vi "Grid_Monitor_V2backupwhite.vi"(7 "Stop (In)":refnum<notifier>, 8 "Error (In)":errorcluster, 11 "SCADA AugState (In)":refnum<notifier>) -> (0 "Error (Out)":errorcluster, 3 "SCADA AugState (Out)":refnum<notifier>, 6 "Stop (Out)":refnum<notifier>)   [LabVIEW 2021]
uses:
  SCADA/SCADA Augmented State.ctl
  Interval.ctl
  SCADA/SCADA Augmented State GUPTA.ctl
  <vilib>/Utility/miscctls.llb/LVForegroundBackgroundColorsTypeDef.ctl
panel:
  out "kW":dbl caption="Numeric" format="%#.3g"
  out "?VkVAr":dbl caption="Numeric" format="%.3g"
  out "A":dbl[unit] caption="Numeric" format="%-^#10.3g"
  out "kW":dbl caption="Numeric" format="%#.3g"
  out "?VkVAr":dbl caption="Numeric" format="%.3g"
  out "A":dbl[unit] caption="Numeric" format="%-^#10.3g"
  out "kW":dbl caption="Numeric" format="%#.3g"
  out "?VkVAr":dbl caption="Numeric" format="%.3g"
  out "A":dbl[unit] caption="Numeric" format="%-^#10.3g"
  out "kW":dbl caption="Numeric" format="%#.3g"
  out "?VkVAr":dbl caption="Numeric" format="%.3g"
  out "A":dbl[unit] caption="Numeric" format="%-^#10.3g"
  out "kW":dbl caption="Numeric" format="%#.3g"
  out "?VkVAr":dbl caption="Numeric" format="%.3g"
  out "A":dbl[unit] caption="Numeric" format="%-^#10.3g"
  out "kW":dbl caption="Numeric" format="%#.3g"
  out "?VkVAr":dbl caption="Numeric" format="%.3g"
  out "A":dbl[unit] caption="Numeric" format="%-^#10.3g"
  out "kW":dbl caption="Numeric" format="%#.3g"
  out "?VkVAr":dbl caption="Numeric" format="%.3g"
  out "A":dbl[unit] caption="Numeric" format="%-^#10.3g"
  out "kW":dbl caption="Numeric" format="%#.3g"
  out "?VkVAr":dbl caption="Numeric" format="%.3g"
  out "A":dbl[unit] caption="Numeric" format="%-^#10.3g"
  out "A":dbl caption="Numeric" format="%-^#10.3g"
  out "kW":dbl caption="Numeric" format="%#.3g"
  out "A":dbl caption="Numeric" format="%-^#10.3g"
  out "kW":dbl caption="Numeric" format="%#.3g"
  out "A":dbl caption="Numeric" format="%-^#10.3g"
  out "kW":dbl caption="Numeric" format="%#.3g"
  out "A":dbl caption="Numeric" format="%-^#10.3g"
  out "kW":dbl caption="Numeric" format="%#.3g"
  out "V slider 11":T1(slide) caption="V-i" scale=230.0..240.0 scale format="%#_4g"
  out "V slider 25":dbl(slide) caption="V-i" max=-10.0 scale=720.0..750.0 scale format="%#_4g"
  out "V slider 24":dbl(slide) caption="V-i" max=-10.0 scale=720.0..750.0 scale format="%#_4g"
  out "V slider 23":dbl(slide) caption="V-i" max=-10.0 scale=720.0..750.0 scale format="%#_4g"
  out "V slider 22":dbl(slide) caption="V-i" max=-10.0 scale=720.0..750.0 scale format="%#_4g"
  out "V slider 21":dbl(slide) caption="V-i" max=-10.0 scale=720.0..750.0 scale format="%#_4g"
  out "V slider 20":dbl(slide) caption="V-i" max=-10.0 scale=720.0..750.0 scale format="%#_4g"
  out "V slider 19":dbl(slide) caption="V-i" max=-10.0 scale=720.0..750.0 scale format="%#_4g"
  out "V slider 18":dbl(slide) caption="V-i" max=-10.0 scale=720.0..750.0 scale format="%#_4g"
  out "V slider 17":T1(slide) caption="V-i" scale=230.0..240.0 scale format="%#_4g"
  out "V slider 16":T1(slide) caption="V-i" scale=230.0..240.0 scale format="%#_4g"
  out "V slider 15":T1(slide) caption="V-i" scale=230.0..240.0 scale format="%#_4g"
  out "V slider 14":T1(slide) caption="V-i" scale=230.0..240.0 scale format="%#_4g"
  out "V slider 13":T1(slide) caption="V-i" scale=230.0..240.0 scale format="%#_4g"
  out "V slider 12":T1(slide) caption="V-i" scale=230.0..240.0 scale format="%#_4g"
  out "V slider 10":T1(slide) caption="V-i" scale=230.0..240.0 scale format="%#_4g"
  out "V slider 9":T1(slide) caption="V-i" scale=230.0..240.0 scale format="%#_4g"
  out "V slider 8":T1(slide) caption="V-i" scale=230.0..240.0 scale format="%#_4g"
  out "V slider 7":T1(slide) caption="V-i" scale=230.0..240.0 scale format="%#_4g"
  out "V slider 6":T1(slide) caption="V-i" scale=230.0..240.0 scale format="%#_4g"
  out "V slider 4":T1(slide) caption="V-i" scale=230.0..240.0 scale format="%#_4g"
  out "V slider 3":T1(slide) caption="V-i" scale=230.0..240.0 scale format="%#_4g"
  out "V slider 1":T1(slide) caption="V-i" scale=230.0..240.0 scale format="%#_4g"
  out "V slider 0":T1(slide) caption="V-i" scale=230.0..240.0 scale format="%#_4g"
  out "I slider 20":dbl(slide) min=-10.0 max=100.0 scale=0.0..100.0
  out "I slider 19":dbl(slide) min=-10.0 max=100.0 scale=0.0..100.0
  out "I slider 18":dbl(slide) min=-10.0 max=100.0 scale=0.0..100.0
  out "I slider 17":dbl(slide) min=-10.0 max=100.0 scale=0.0..100.0
  out "I slider 16":T1(slide) scale=0.0..44.0
  out "I slider 15":T1(slide) scale=0.0..44.0
  out "I slider 14":T1(slide) scale=0.0..44.0
  out "I slider 13":T1(slide) scale=0.0..44.0
  out "I slider 12":T1(slide) scale=0.0..108.0
  out "I slider 11":T1(slide) scale=0.0..82.0
  out "I slider 10":T1(slide) scale=0.0..82.0 scale format="%^#1.3g"
  out "I slider 9":T1(slide) scale=0.0..44.0
  out "I slider 8":T1(slide) scale=0.0..82.0 scale format="%^#1.3g"
  out "I slider 7":T1(slide) scale=0.0..207.0
  out "I slider 6":T1(slide) scale=0.0..135.0 scale format="%^#1.3g"
  out "I slider 5":T1(slide) scale=0.0..82.0
  out "I slider 4":T1(slide) scale=0.0..82.0
  out "I slider 3":T1(slide) scale=0.0..108.0
  out "I slider 2":T1(slide) scale=0.0..207.0 scale format="%^#1.3g"
  out "I slider 0":T1(slide) scale=0.0..207.0
  out "I slider 1":T1(slide) scale=0.0..44.0
  out "V slider 2":T1(slide) caption="V-i" scale=230.0..240.0 scale format="%#_4g"
  out "A":dbl caption="Numeric" format="%-^#10.3g"
  out "kW":dbl caption="Numeric" format="%#.3g"
  out "A":dbl caption="Numeric" format="%-^#10.3g"
  out "kW":dbl caption="Numeric" format="%#.3g"
  out "A":dbl caption="Numeric" format="%-^#10.3g"
  out "kW":dbl caption="Numeric" format="%#.3g"
  out "A":dbl[unit] caption="Numeric" format="%-^#10.3g"
  out "?VkVAr":dbl caption="Numeric" format="%.3g"
  out "kW":dbl caption="Numeric" format="%#.3g"
  out "A":dbl[unit] caption="Numeric" format="%-^#10.3g"
  out "?VkVAr":dbl caption="Numeric" format="%.3g"
  out "kW":dbl caption="Numeric" format="%#.3g"
  in  "Stop?":bool
  out "Connected?":bool
  out "AugState (Out)":refnum<notifier>
  in  "AugState (In)":refnum<notifier>
  # "EL"
  # "L"
  # "Electrolyzer"
  # "Load"
  # "FC"
  # "B"
  # "Fuel Cell"
  # "Battery"
  # "PV"
  # "SC"
  # "Photovoltaic"
  # "Super Caps"
  # "V"
  # "B03"
  # "B01"
  # "PMU locations"
  # "DMU locations"
  # "B02"
  # "1"
  # "9"
  # "2"
  # "B05"
  # "B07"
  # "B14"
  # "B04"
  # "B06"
  # "7"
  # "3"
  # "A"
  # "B18"
  # "B22"
  # "B26"
  # "4"
  # "8"
  # "10"
  # "A"
  # "B09"
  # "B08"
  # "B17"
  # "B21"
  # "B25"
  # "4"
  # "3"
  # "7"
  # "11"
  # "B11"
  # "B16"
  # "B20"
  # "B24"
  # "B10"
  # "5"
  # "2"
  # "6"
  # "12"
  # "B13"
  # "B12"
  # "6"
  # "B15"
  # "B19"
  # "B23"
  # "1"
  # "5"
  # "13"
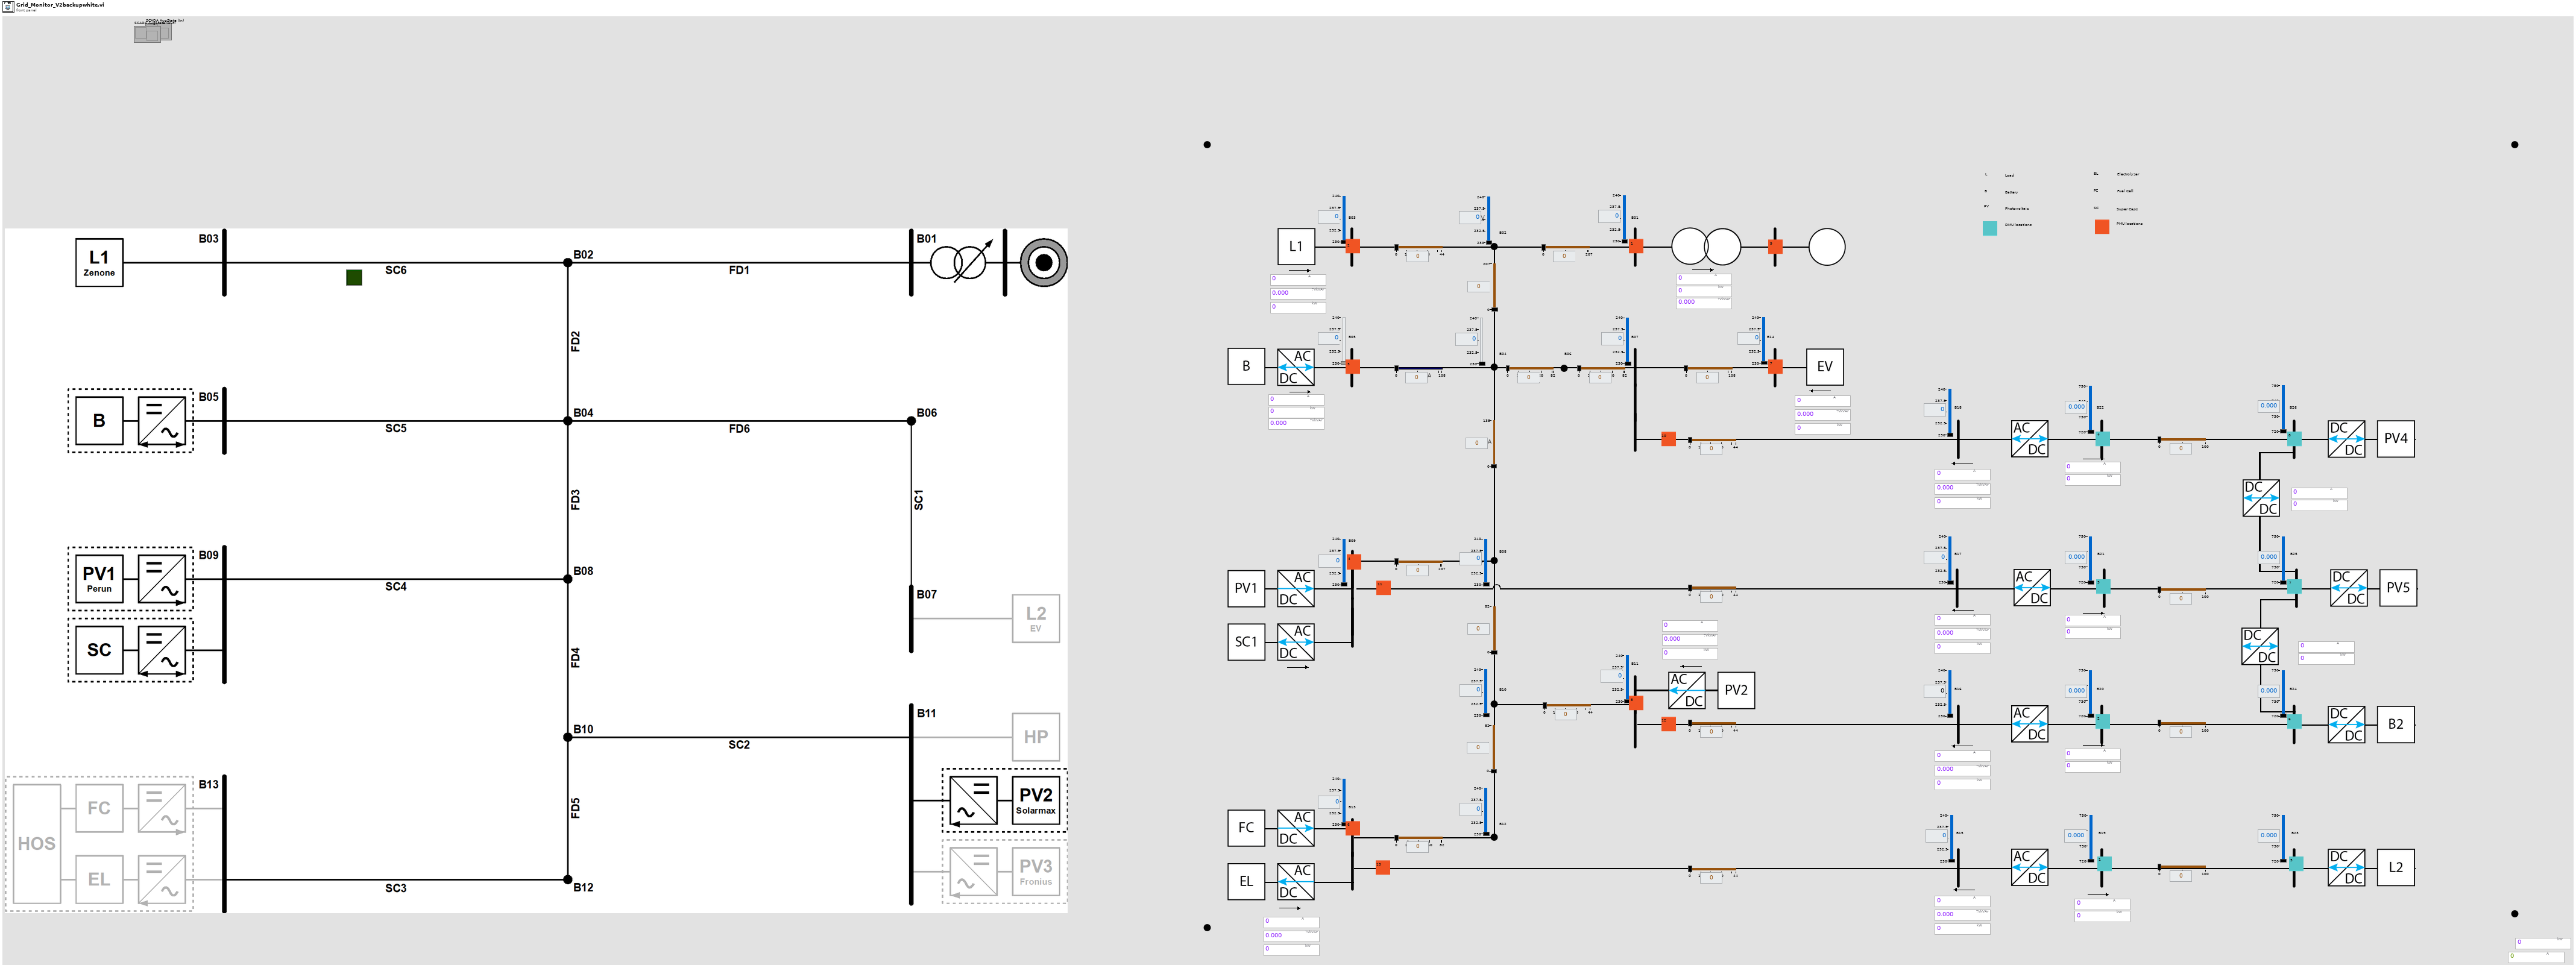
[diagram p1: front panel]
types:
  T1 = cluster{"Numeric":dbl, "Numeric":dbl, "Numeric":dbl}
  T2 = typedef "LVForegroundBackgroundColorsTypeDef.ctl" = cluster{"Foreground Color":u32, "Background Color":u32}
  T3 = typedef "SCADA Augmented State GUPTA.ctl" = cluster{"Buses":cluster{"Vbus":cdb[], "Iinjected":cdb[], "Sinjected":cdb[], "Vband":T4}[], "Lines":cluster{"Iforward":cdb[], "Ibackward":cdb[], "Imaximum":dbl}[], "f_downstream":dbl, "V_upstream":cdb[], "f_upstream":dbl, "Timestamp":timestamp, "M ":cluster{cdb, cdb, cdb}[], "z(k|k)":dbl[], "r(k)":dbl[], "Arrival (SE)":timestamp, "Arrival (PDC)":timestamp, "Departure (SE)":timestamp, "T":dbl[]}
  T4 = typedef "Interval.ctl" = cluster{"lower":dbl, "upper":dbl}
  T5 = cluster{"Iforward":cdb[], "Ibackward":cdb[], "Imaximum":dbl}[]
  T6 = cluster{"Vbus":cdb[], "Iinjected":cdb[], "Sinjected":cdb[], "Vband":T4}[]
  T7 = cluster{"Vbus":cdb[], "Iinjected":cdb[], "Sinjected":cdb[], "Vband":T4}
  T8 = cluster{"I_trip":dbl, "Phasor C":dbl, "Phasor C":dbl, "Phasor C":dbl}
  T9 = cluster{"V_maximum":dbl, "Phasor C":dbl, "Phasor C":dbl, "Phasor C":dbl, "V_minimun":dbl}
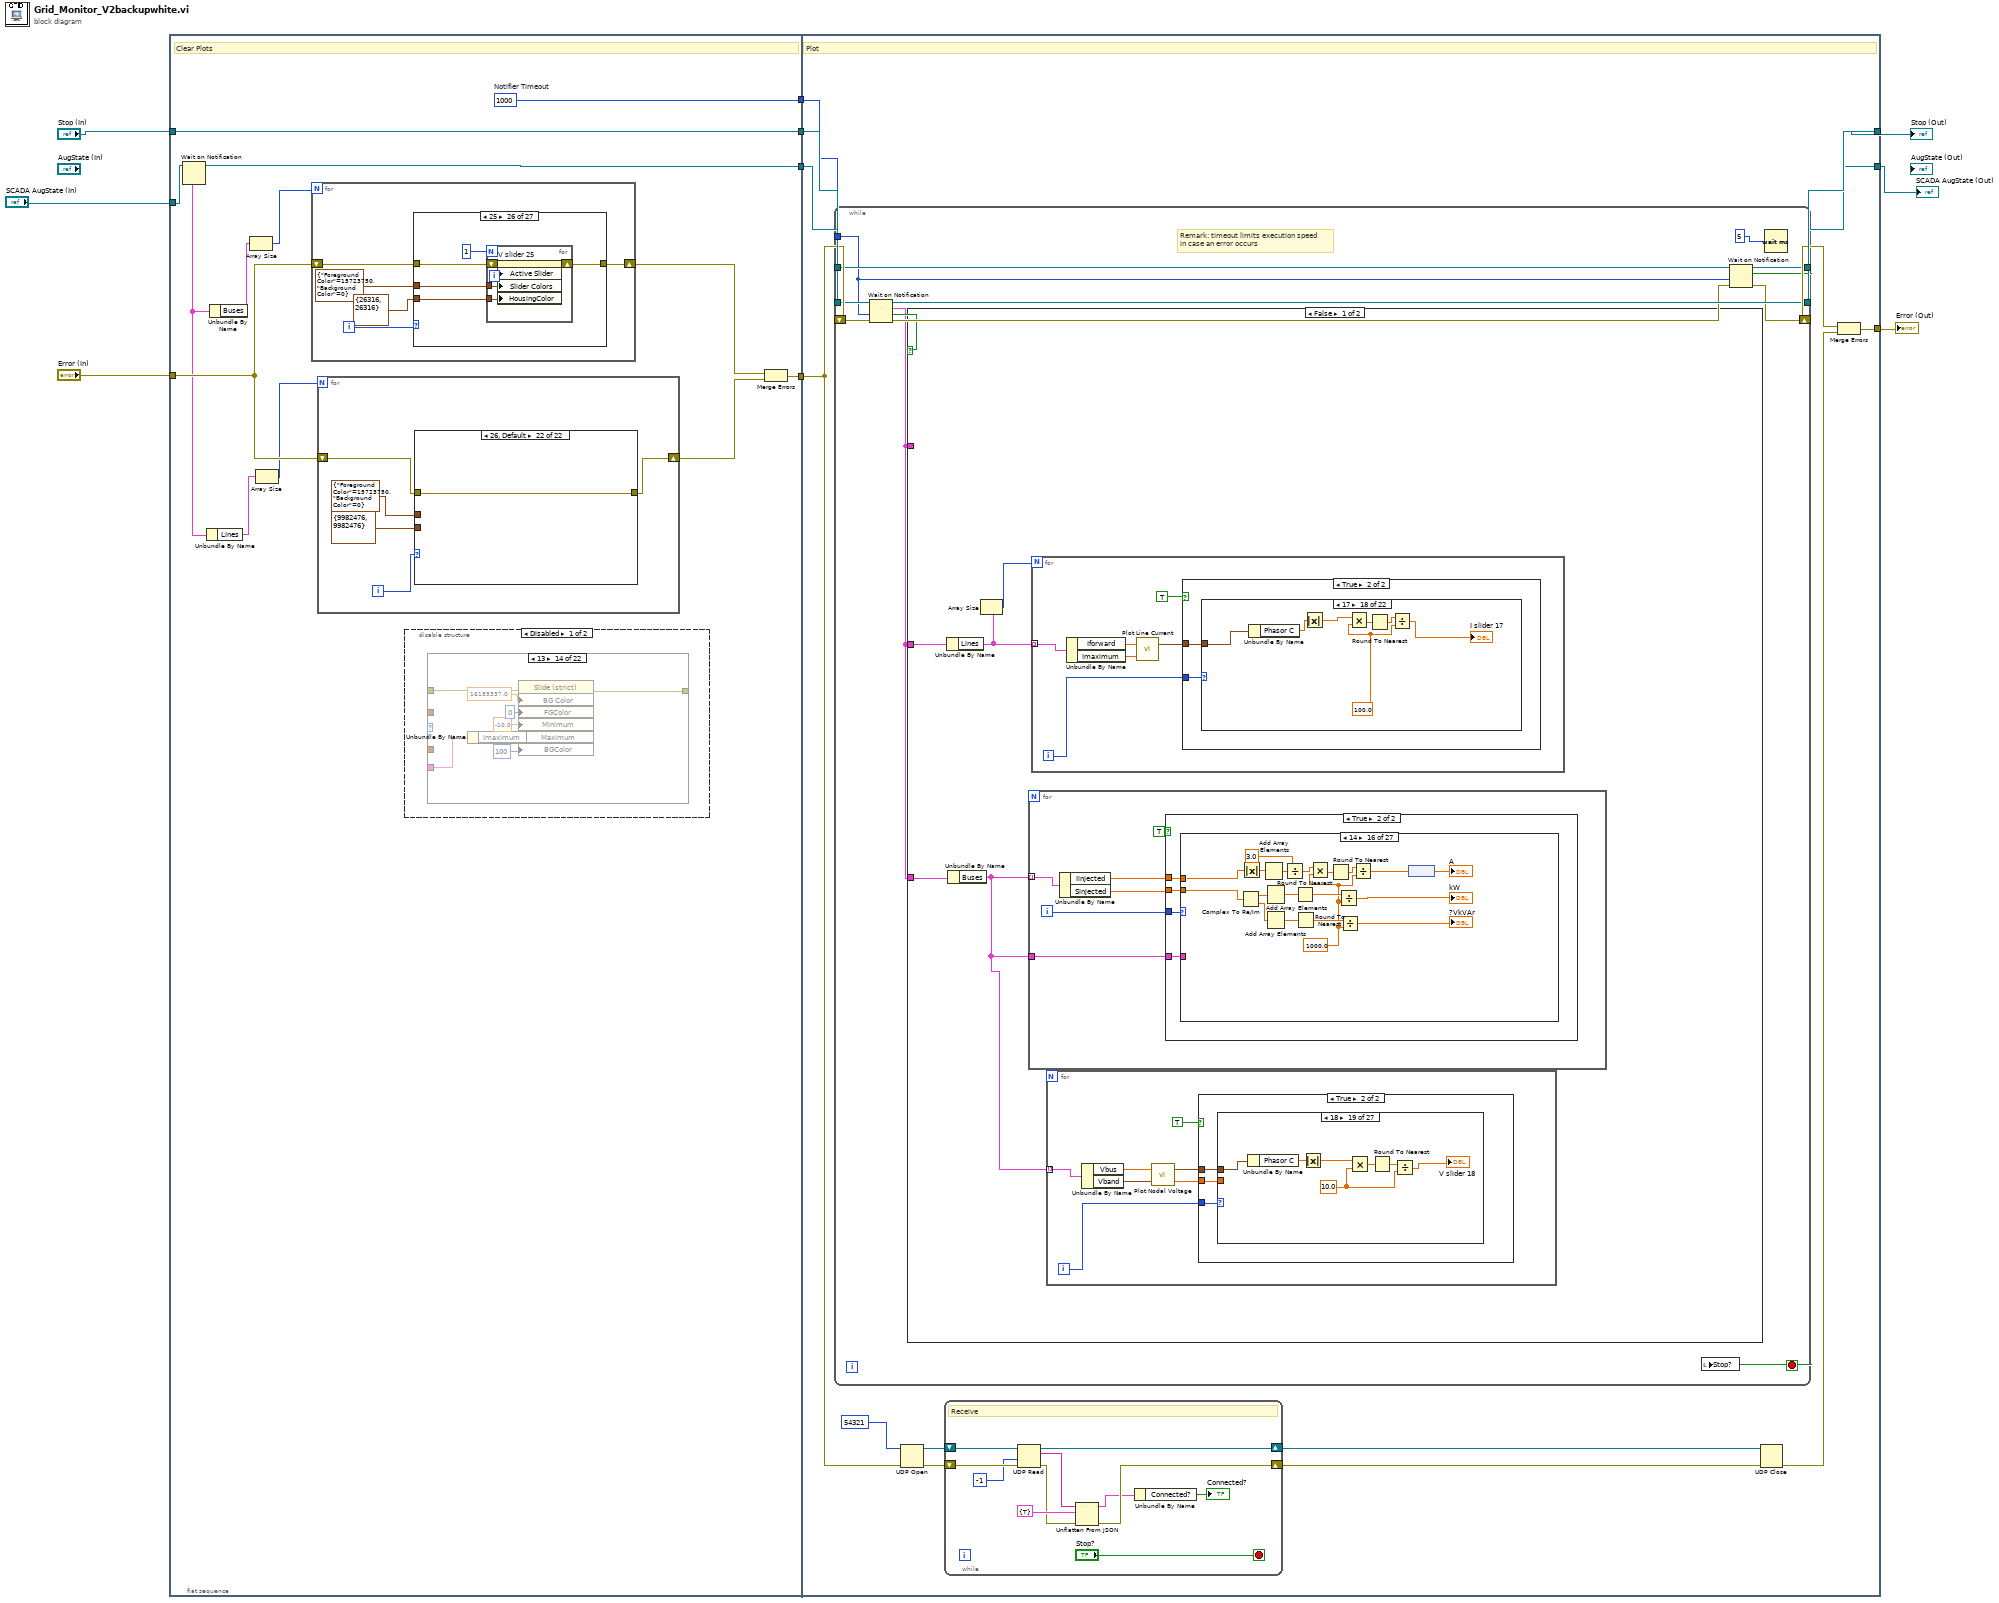
[diagram p0: block diagram]
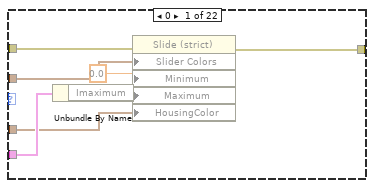
[diagram p2: hidden frame]
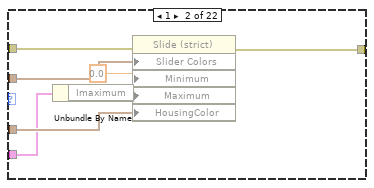
[diagram p3: hidden frame]
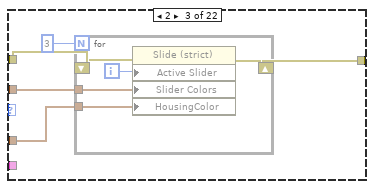
[diagram p4: hidden frame]
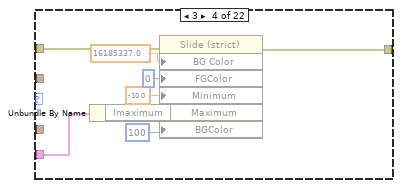
[diagram p5: hidden frame]
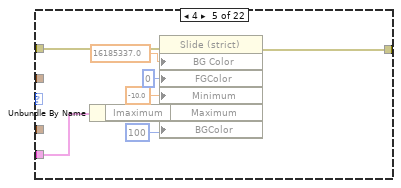
[diagram p6: hidden frame]
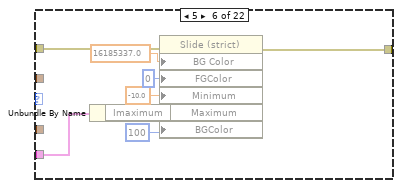
[diagram p7: hidden frame]
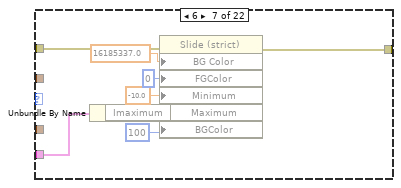
[diagram p8: hidden frame]
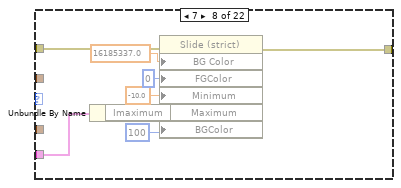
[diagram p9: hidden frame]
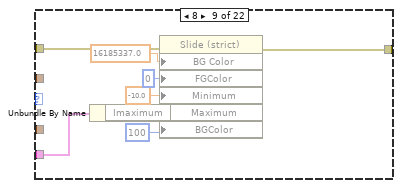
[diagram p10: hidden frame]
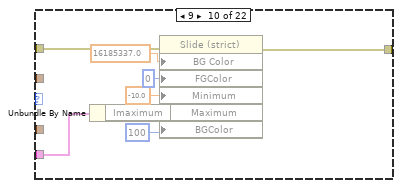
[diagram p11: hidden frame]
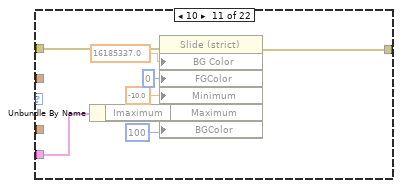
[diagram p12: hidden frame]
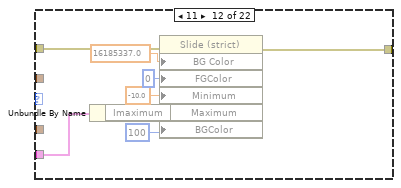
[diagram p13: hidden frame]
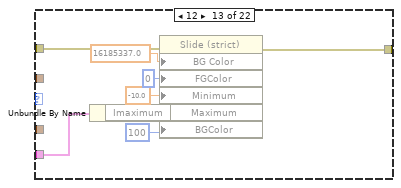
[diagram p14: hidden frame]
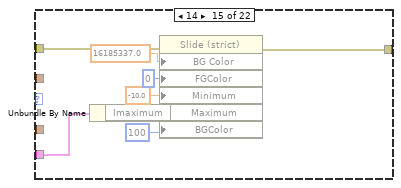
[diagram p15: hidden frame]
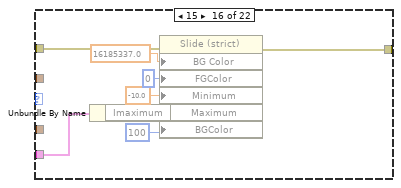
[diagram p16: hidden frame]
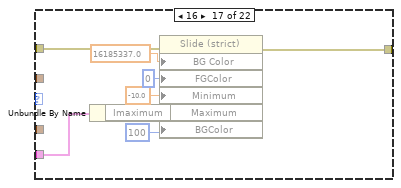
[diagram p17: hidden frame]
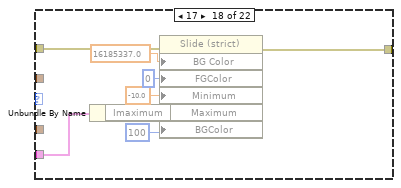
[diagram p18: hidden frame]
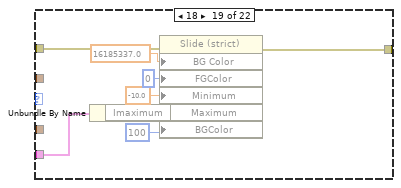
[diagram p19: hidden frame]
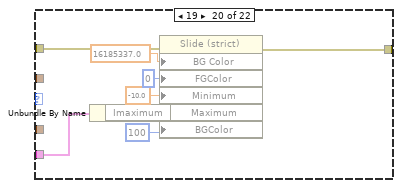
[diagram p20: hidden frame]
diagram:
  n1 = flat-sequence {
    tunnel: "Stop (In)" -> [w23]
    tunnel: [w16] -> w8
    tunnel: [w23] -> w7
    tunnel: [w20] -> w6
    tunnel: "Error (In)" -> [w19]
    tunnel: [w18] -> w3
    tunnel: "SCADA AugState (In)" -> [w17]
    tunnel: [w677] -> w9
    tunnel: [w668] -> w4
    tunnel: w8 -> [w679]
    tunnel: w7 -> [w678]
    tunnel: w6 -> [w670]
    tunnel: w3 -> [w676]
    tunnel: [w666] -> w2
    frame #0 {
      w18 = 1000  # Notifier Timeout
      # "Clear Plots"
      n2 = Wait on Notification(notifier=w17) -> (notifier out=w16:refnum<notifier>, notification=w14:T3)  [unwired: 3 in, 2 out]
      n3 = Unbundle By Name(w14) -> ("Lines"=w11:T5)
      n4 = Unbundle By Name(w14) -> ("Buses"=w13:T6)
      n5 = Array Size(array=w13) -> (size(s)=w12:i32)
      n6 = Array Size(array=w11) -> (size(s)=w15:i32)
      n7 = for {
        N: w12 -> [_]
        shift-right: [w409] -> w22
        shift-left: w19 -> [w411]
        i -> [w410]
        n8 = case shown="25" w410 {
          tunnel: w411 -> [w415 w425 w435 w444 w453 w462 w468 w478 w488 w498 w508 w518 w528 w538 w548 w558 w568 w578 w588 w598 w608 w618 w628 w638 w648 w658 w665]
          tunnel: [w416 w426 w436 w445 w454 w463 w469 w479 w489 w499 w509 w519 w529 w539 w549 w559 w569 w579 w589 w599 w609 w619 w629 w639 w649 w659 w665] -> w409
          tunnel: T2 {"Foreground Color"=15723750, "Background Color"=0} ("Slider Colors") -> [w413 w423 w433 w442 w451 w460 w466 w476 w486 w496 w506 w516 w526 w536 w546 w556 w566 w576 w586 w596 w606 w616 w626 w636 w646 w656 _]
          tunnel: T2 {"Foreground Color"=26316, "Background Color"=26316} ("Slider Colors") -> [w412 w422 w432 _ w450 _ w465 w475 w485 w495 w505 w515 w525 w535 w545 w555 w565 w575 w585 w595 w605 w615 w625 w635 w645 w655 _]
          frame 0 {
            n9 = for {
              N: 3 -> [_]
              tunnel: w413 -> [w419]
              shift-right: [w421] -> w416
              shift-left: w415 -> [w420]
              tunnel: w412 -> [w417]
              i -> [w418]
              n10 = property on="V slider 0" class="Slide (strict)"(error in=w420, "Active Slider"=w418, "Slider Colors"=w419, "HousingColor"=w417) -> (error out=w421:errorcluster)  [unwired: 1 in, 1 out]
            }
          }
          frame 1 {
            n11 = for {
              N: 3 -> [_]
              tunnel: w423 -> [w429]
              shift-right: [w431] -> w426
              shift-left: w425 -> [w430]
              tunnel: w422 -> [w427]
              i -> [w428]
              n12 = property on="V slider 1" class="Slide (strict)"(error in=w430, "Active Slider"=w428, "Slider Colors"=w429, "HousingColor"=w427) -> (error out=w431:errorcluster)  [unwired: 1 in, 1 out]
            }
          }
          frame 2 {
            n13 = for {
              N: 3 -> [_]
              tunnel: w433 -> [w439]
              shift-right: [w441] -> w436
              shift-left: w435 -> [w440]
              tunnel: w432 -> [w437]
              i -> [w438]
              n14 = property on="V slider 2" class="Slide (strict)"(error in=w440, "Active Slider"=w438, "Slider Colors"=w439, "HousingColor"=w437) -> (error out=w441:errorcluster)  [unwired: 1 in, 1 out]
            }
          }
          frame 3 {
            n15 = for {
              N: 3 -> [_]
              tunnel: w442 -> [w447]
              shift-right: [w449] -> w445
              shift-left: w444 -> [w448]
              i -> [w446]
              n16 = property on="V slider 3" class="Slide (strict)"(error in=w448, "Active Slider"=w446, "Slider Colors"=w447) -> (error out=w449:errorcluster)  [unwired: 1 in, 1 out]
            }
          }
          frame 4 {
            n17 = for {
              N: 3 -> [_]
              tunnel: w451 -> [w457]
              shift-right: [w459] -> w454
              shift-left: w453 -> [w458]
              tunnel: w450 -> [w455]
              i -> [w456]
              n18 = property on="I slider 4" class="Slide (strict)"(error in=w458, "Active Slider"=w456, "Slider Colors"=w457, "HousingColor"=w455) -> (error out=w459:errorcluster)  [unwired: 1 in, 1 out]
            }
          }
          frame 5 {
            n19 = for {
              N: 3 -> [_]
              tunnel: w460 -> [_]
              shift-right: [w464] -> w463
              shift-left: w462 -> [w464]
            }
          }
          frame 6 {
            n20 = for {
              N: 3 -> [_]
              tunnel: w466 -> [w472]
              shift-right: [w474] -> w469
              shift-left: w468 -> [w473]
              tunnel: w465 -> [w470]
              i -> [w471]
              n21 = property on="V slider 6" class="Slide (strict)"(error in=w473, "Active Slider"=w471, "Slider Colors"=w472, "HousingColor"=w470) -> (error out=w474:errorcluster)  [unwired: 1 in, 1 out]
            }
          }
          frame 7 {
            n22 = for {
              N: 3 -> [_]
              tunnel: w476 -> [w482]
              shift-right: [w484] -> w479
              shift-left: w478 -> [w483]
              tunnel: w475 -> [w480]
              i -> [w481]
              n23 = property on="V slider 7" class="Slide (strict)"(error in=w483, "Active Slider"=w481, "Slider Colors"=w482, "HousingColor"=w480) -> (error out=w484:errorcluster)  [unwired: 1 in, 1 out]
            }
          }
          frame 8 {
            n24 = for {
              N: 3 -> [_]
              tunnel: w486 -> [w492]
              shift-right: [w494] -> w489
              shift-left: w488 -> [w493]
              tunnel: w485 -> [w490]
              i -> [w491]
              n25 = property on="V slider 8" class="Slide (strict)"(error in=w493, "Active Slider"=w491, "Slider Colors"=w492, "HousingColor"=w490) -> (error out=w494:errorcluster)  [unwired: 1 in, 1 out]
            }
          }
          frame 9 {
            n26 = for {
              N: 3 -> [_]
              tunnel: w496 -> [w502]
              shift-right: [w504] -> w499
              shift-left: w498 -> [w503]
              tunnel: w495 -> [w500]
              i -> [w501]
              n27 = property on="V slider 9" class="Slide (strict)"(error in=w503, "Active Slider"=w501, "Slider Colors"=w502, "HousingColor"=w500) -> (error out=w504:errorcluster)  [unwired: 1 in, 1 out]
            }
          }
          frame 10 {
            n28 = for {
              N: 3 -> [_]
              tunnel: w506 -> [w512]
              shift-right: [w514] -> w509
              shift-left: w508 -> [w513]
              tunnel: w505 -> [w510]
              i -> [w511]
              n29 = property on="V slider 10" class="Slide (strict)"(error in=w513, "Active Slider"=w511, "Slider Colors"=w512, "HousingColor"=w510) -> (error out=w514:errorcluster)  [unwired: 1 in, 1 out]
            }
          }
          frame 11 {
            n30 = for {
              N: 3 -> [_]
              tunnel: w516 -> [w521]
              shift-right: [w523] -> w519
              shift-left: w518 -> [w524]
              tunnel: w515 -> [w520]
              i -> [w522]
              n31 = property on="V slider 11" class="Slide (strict)"(error in=w524, "Active Slider"=w522, "Slider Colors"=w521, "HousingColor"=w520) -> (error out=w523:errorcluster)  [unwired: 1 in, 1 out]
            }
          }
          frame 12 {
            n32 = for {
              N: 3 -> [_]
              tunnel: w526 -> [w532]
              shift-right: [w534] -> w529
              shift-left: w528 -> [w533]
              tunnel: w525 -> [w530]
              i -> [w531]
              n33 = property on="V slider 12" class="Slide (strict)"(error in=w533, "Active Slider"=w531, "Slider Colors"=w532, "HousingColor"=w530) -> (error out=w534:errorcluster)  [unwired: 1 in, 1 out]
            }
          }
          frame 13 {
            n34 = for {
              N: 3 -> [_]
              tunnel: w536 -> [w542]
              shift-right: [w544] -> w539
              shift-left: w538 -> [w543]
              tunnel: w535 -> [w540]
              i -> [w541]
              n35 = property on="V slider 13" class="Slide (strict)"(error in=w543, "Active Slider"=w541, "Slider Colors"=w542, "HousingColor"=w540) -> (error out=w544:errorcluster)  [unwired: 1 in, 1 out]
            }
          }
          frame 14 {
            n36 = for {
              N: 3 -> [_]
              tunnel: w546 -> [w552]
              shift-right: [w554] -> w549
              shift-left: w548 -> [w553]
              tunnel: w545 -> [w550]
              i -> [w551]
              n37 = property on="V slider 14" class="Slide (strict)"(error in=w553, "Active Slider"=w551, "Slider Colors"=w552, "HousingColor"=w550) -> (error out=w554:errorcluster)  [unwired: 1 in, 1 out]
            }
          }
          frame 15 {
            n38 = for {
              N: 3 -> [_]
              tunnel: w556 -> [w562]
              shift-right: [w564] -> w559
              shift-left: w558 -> [w563]
              tunnel: w555 -> [w560]
              i -> [w561]
              n39 = property on="V slider 15" class="Slide (strict)"(error in=w563, "Active Slider"=w561, "Slider Colors"=w562, "HousingColor"=w560) -> (error out=w564:errorcluster)  [unwired: 1 in, 1 out]
            }
          }
          frame 16 {
            n40 = for {
              N: 3 -> [_]
              tunnel: w566 -> [w572]
              shift-right: [w574] -> w569
              shift-left: w568 -> [w573]
              tunnel: w565 -> [w570]
              i -> [w571]
              n41 = property on="V slider 16" class="Slide (strict)"(error in=w573, "Active Slider"=w571, "Slider Colors"=w572, "HousingColor"=w570) -> (error out=w574:errorcluster)  [unwired: 1 in, 1 out]
            }
          }
          frame 17 {
            n42 = for {
              N: 3 -> [_]
              tunnel: w576 -> [w582]
              shift-right: [w584] -> w579
              shift-left: w578 -> [w583]
              tunnel: w575 -> [w580]
              i -> [w581]
              n43 = property on="V slider 17" class="Slide (strict)"(error in=w583, "Active Slider"=w581, "Slider Colors"=w582, "HousingColor"=w580) -> (error out=w584:errorcluster)  [unwired: 1 in, 1 out]
            }
          }
          frame 18 {
            n44 = for {
              N: 1 -> [_]
              shift-right: [w594] -> w589
              shift-left: w588 -> [w593]
              tunnel: w586 -> [w591]
              tunnel: w585 -> [w590]
              i -> [w592]
              n45 = property on="V slider 18" class="Slide (strict)"(error in=w593, "Active Slider"=w592, "Slider Colors"=w591, "HousingColor"=w590) -> (error out=w594:errorcluster)  [unwired: 1 in, 1 out]
            }
          }
          frame 19 {
            n46 = for {
              N: 1 -> [_]
              tunnel: w596 -> [w602]
              shift-right: [w604] -> w599
              shift-left: w598 -> [w603]
              tunnel: w595 -> [w600]
              i -> [w601]
              n47 = property on="V slider 19" class="Slide (strict)"(error in=w603, "Active Slider"=w601, "Slider Colors"=w602, "HousingColor"=w600) -> (error out=w604:errorcluster)  [unwired: 1 in, 1 out]
            }
          }
          frame 20 {
            n48 = for {
              N: 1 -> [_]
              tunnel: w606 -> [w612]
              shift-right: [w614] -> w609
              shift-left: w608 -> [w613]
              tunnel: w605 -> [w610]
              i -> [w611]
              n49 = property on="V slider 20" class="Slide (strict)"(error in=w613, "Active Slider"=w611, "Slider Colors"=w612, "HousingColor"=w610) -> (error out=w614:errorcluster)  [unwired: 1 in, 1 out]
            }
          }
          frame 21 {
            n50 = for {
              N: 1 -> [_]
              tunnel: w616 -> [w622]
              shift-right: [w624] -> w619
              shift-left: w618 -> [w623]
              tunnel: w615 -> [w620]
              i -> [w621]
              n51 = property on="V slider 21" class="Slide (strict)"(error in=w623, "Active Slider"=w621, "Slider Colors"=w622, "HousingColor"=w620) -> (error out=w624:errorcluster)  [unwired: 1 in, 1 out]
            }
          }
          frame 22 {
            n52 = for {
              N: 1 -> [_]
              tunnel: w626 -> [w632]
              shift-right: [w634] -> w629
              shift-left: w628 -> [w633]
              tunnel: w625 -> [w630]
              i -> [w631]
              n53 = property on="V slider 22" class="Slide (strict)"(error in=w633, "Active Slider"=w631, "Slider Colors"=w632, "HousingColor"=w630) -> (error out=w634:errorcluster)  [unwired: 1 in, 1 out]
            }
          }
          frame 23 {
            n54 = for {
              N: 1 -> [_]
              tunnel: w636 -> [w642]
              shift-right: [w644] -> w639
              shift-left: w638 -> [w643]
              tunnel: w635 -> [w640]
              i -> [w641]
              n55 = property on="V slider 23" class="Slide (strict)"(error in=w643, "Active Slider"=w641, "Slider Colors"=w642, "HousingColor"=w640) -> (error out=w644:errorcluster)  [unwired: 1 in, 1 out]
            }
          }
          frame 24 {
            n56 = for {
              N: 1 -> [_]
              tunnel: w646 -> [w652]
              shift-right: [w654] -> w649
              shift-left: w648 -> [w653]
              tunnel: w645 -> [w650]
              i -> [w651]
              n57 = property on="V slider 24" class="Slide (strict)"(error in=w653, "Active Slider"=w651, "Slider Colors"=w652, "HousingColor"=w650) -> (error out=w654:errorcluster)  [unwired: 1 in, 1 out]
            }
          }
          frame 25 {
            n58 = for {
              N: 1 -> [_]
              tunnel: w656 -> [w662]
              shift-right: [w664] -> w659
              shift-left: w658 -> [w663]
              tunnel: w655 -> [w660]
              i -> [w661]
              n59 = property on="V slider 25" class="Slide (strict)"(error in=w663, "Active Slider"=w661, "Slider Colors"=w662, "HousingColor"=w660) -> (error out=w664:errorcluster)  [unwired: 1 in, 1 out]
            }
          }
          frame 26, Default {
          }
        }
      }
      n60 = for {
        N: w15 -> [_]
        shift-right: [w193] -> w21
        shift-left: w19 -> [w194]
        i -> [w197]
        n61 = case shown="26, Default" w197 {
          tunnel: w194 -> [w201 w211 w221 w230 w239 w246 w259 w269 w279 w289 w299 w309 w319 w329 w339 w349 w359 w369 w379 w389 w399 w406]
          tunnel: [w202 w212 w222 w231 w240 w249 w260 w270 w280 w290 w300 w310 w320 w330 w340 w350 w360 w370 w380 w390 w400 w406] -> w193
          tunnel: T2 {"Foreground Color"=15723750, "Background Color"=0} ("Slider Colors") -> [w199 w209 w219 w228 w237 w247 w257 w267 w277 w287 w297 w307 w317 w327 w337 w347 w357 w367 w377 w387 w397 _]
          tunnel: T2 {"Foreground Color"=9982476, "Background Color"=9982476} ("Slider Colors") -> [w198 w208 w218 _ w236 w248 w256 w266 w276 w286 w296 w306 w316 w326 w336 w346 w356 w366 w376 w386 w396 _]
          frame 0 {
            n62 = for {
              N: 3 -> [_]
              tunnel: w199 -> [w205]
              shift-right: [w207] -> w202
              shift-left: w201 -> [w206]
              tunnel: w198 -> [w203]
              i -> [w204]
              n63 = property on="I slider 0" class="Slide (strict)"(error in=w206, "Active Slider"=w204, "Slider Colors"=w205, "HousingColor"=w203) -> (error out=w207:errorcluster)  [unwired: 1 in, 1 out]
            }
          }
          frame 1 {
            n64 = for {
              N: 3 -> [_]
              tunnel: w209 -> [w215]
              shift-right: [w217] -> w212
              shift-left: w211 -> [w216]
              tunnel: w208 -> [w213]
              i -> [w214]
              n65 = property on="I slider 1" class="Slide (strict)"(error in=w216, "Active Slider"=w214, "Slider Colors"=w215, "HousingColor"=w213) -> (error out=w217:errorcluster)  [unwired: 1 in, 1 out]
            }
          }
          frame 2 {
            n66 = for {
              N: 3 -> [_]
              tunnel: w219 -> [w225]
              shift-right: [w227] -> w222
              shift-left: w221 -> [w226]
              tunnel: w218 -> [w223]
              i -> [w224]
              n67 = property on="I slider 2" class="Slide (strict)"(error in=w226, "Active Slider"=w224, "Slider Colors"=w225, "HousingColor"=w223) -> (error out=w227:errorcluster)  [unwired: 1 in, 1 out]
            }
          }
          frame 3 {
            n68 = for {
              N: 3 -> [_]
              tunnel: w228 -> [w233]
              shift-right: [w235] -> w231
              shift-left: w230 -> [w234]
              i -> [w232]
              n69 = property on="I slider 3" class="Slide (strict)"(error in=w234, "Active Slider"=w232, "Slider Colors"=w233) -> (error out=w235:errorcluster)  [unwired: 1 in, 1 out]
            }
          }
          frame 4 {
            n70 = for {
              N: 3 -> [_]
              tunnel: w237 -> [w243]
              shift-right: [w245] -> w240
              shift-left: w239 -> [w244]
              tunnel: w236 -> [w241]
              i -> [w242]
              n71 = property on="I slider 4" class="Slide (strict)"(error in=w244, "Active Slider"=w242, "Slider Colors"=w243, "HousingColor"=w241) -> (error out=w245:errorcluster)  [unwired: 1 in, 1 out]
            }
          }
          frame 5 {
            n72 = for {
              N: 3 -> [_]
              tunnel: w247 -> [w253]
              shift-right: [w255] -> w249
              shift-left: w246 -> [w254]
              tunnel: w248 -> [w251]
              i -> [w252]
              n73 = property on="I slider 5" class="Slide (strict)"(error in=w254, "Active Slider"=w252, "Slider Colors"=w253, "HousingColor"=w251) -> (error out=w255:errorcluster)  [unwired: 1 in, 1 out]
            }
          }
          frame 6 {
            n74 = for {
              N: 3 -> [_]
              tunnel: w257 -> [w263]
              shift-right: [w265] -> w260
              shift-left: w259 -> [w264]
              tunnel: w256 -> [w261]
              i -> [w262]
              n75 = property on="I slider 6" class="Slide (strict)"(error in=w264, "Active Slider"=w262, "Slider Colors"=w263, "HousingColor"=w261) -> (error out=w265:errorcluster)  [unwired: 1 in, 1 out]
            }
          }
          frame 7 {
            n76 = for {
              N: 3 -> [_]
              tunnel: w267 -> [w273]
              shift-right: [w275] -> w270
              shift-left: w269 -> [w274]
              tunnel: w266 -> [w271]
              i -> [w272]
              n77 = property on="I slider 7" class="Slide (strict)"(error in=w274, "Active Slider"=w272, "Slider Colors"=w273, "HousingColor"=w271) -> (error out=w275:errorcluster)  [unwired: 1 in, 1 out]
            }
          }
          frame 8 {
            n78 = for {
              N: 3 -> [_]
              tunnel: w277 -> [w283]
              shift-right: [w285] -> w280
              shift-left: w279 -> [w284]
              tunnel: w276 -> [w281]
              i -> [w282]
              n79 = property on="I slider 8" class="Slide (strict)"(error in=w284, "Active Slider"=w282, "Slider Colors"=w283, "HousingColor"=w281) -> (error out=w285:errorcluster)  [unwired: 1 in, 1 out]
            }
          }
          frame 9 {
            n80 = for {
              N: 3 -> [_]
              tunnel: w287 -> [w293]
              shift-right: [w295] -> w290
              shift-left: w289 -> [w294]
              tunnel: w286 -> [w291]
              i -> [w292]
              n81 = property on="I slider 9" class="Slide (strict)"(error in=w294, "Active Slider"=w292, "Slider Colors"=w293, "HousingColor"=w291) -> (error out=w295:errorcluster)  [unwired: 1 in, 1 out]
            }
          }
          frame 10 {
            n82 = for {
              N: 3 -> [_]
              tunnel: w297 -> [w303]
              shift-right: [w305] -> w300
              shift-left: w299 -> [w304]
              tunnel: w296 -> [w301]
              i -> [w302]
              n83 = property on="I slider 10" class="Slide (strict)"(error in=w304, "Active Slider"=w302, "Slider Colors"=w303, "HousingColor"=w301) -> (error out=w305:errorcluster)  [unwired: 1 in, 1 out]
            }
          }
          frame 11 {
            n84 = for {
              N: 3 -> [_]
              tunnel: w307 -> [w312]
              shift-right: [w314] -> w310
              shift-left: w309 -> [w315]
              tunnel: w306 -> [w311]
              i -> [w313]
              n85 = property on="I slider 11" class="Slide (strict)"(error in=w315, "Active Slider"=w313, "Slider Colors"=w312, "HousingColor"=w311) -> (error out=w314:errorcluster)  [unwired: 1 in, 1 out]
            }
          }
          frame 12 {
            n86 = for {
              N: 3 -> [_]
              tunnel: w317 -> [w323]
              shift-right: [w325] -> w320
              shift-left: w319 -> [w324]
              tunnel: w316 -> [w321]
              i -> [w322]
              n87 = property on="I slider 12" class="Slide (strict)"(error in=w324, "Active Slider"=w322, "Slider Colors"=w323, "HousingColor"=w321) -> (error out=w325:errorcluster)  [unwired: 1 in, 1 out]
            }
          }
          frame 13 {
            n88 = for {
              N: 3 -> [_]
              tunnel: w327 -> [w333]
              shift-right: [w335] -> w330
              shift-left: w329 -> [w334]
              tunnel: w326 -> [w331]
              i -> [w332]
              n89 = property on="I slider 13" class="Slide (strict)"(error in=w334, "Active Slider"=w332, "Slider Colors"=w333, "HousingColor"=w331) -> (error out=w335:errorcluster)  [unwired: 1 in, 1 out]
            }
          }
          frame 14 {
            n90 = for {
              N: 3 -> [_]
              tunnel: w337 -> [w343]
              shift-right: [w345] -> w340
              shift-left: w339 -> [w344]
              tunnel: w336 -> [w341]
              i -> [w342]
              n91 = property on="I slider 14" class="Slide (strict)"(error in=w344, "Active Slider"=w342, "Slider Colors"=w343, "HousingColor"=w341) -> (error out=w345:errorcluster)  [unwired: 1 in, 1 out]
            }
          }
          frame 15 {
            n92 = for {
              N: 3 -> [_]
              tunnel: w347 -> [w353]
              shift-right: [w355] -> w350
              shift-left: w349 -> [w354]
              tunnel: w346 -> [w351]
              i -> [w352]
              n93 = property on="I slider 15" class="Slide (strict)"(error in=w354, "Active Slider"=w352, "Slider Colors"=w353, "HousingColor"=w351) -> (error out=w355:errorcluster)  [unwired: 1 in, 1 out]
            }
          }
          frame 16 {
            n94 = for {
              N: 3 -> [_]
              tunnel: w357 -> [w363]
              shift-right: [w365] -> w360
              shift-left: w359 -> [w364]
              tunnel: w356 -> [w361]
              i -> [w362]
              n95 = property on="I slider 16" class="Slide (strict)"(error in=w364, "Active Slider"=w362, "Slider Colors"=w363, "HousingColor"=w361) -> (error out=w365:errorcluster)  [unwired: 1 in, 1 out]
            }
          }
          frame 17 {
            n96 = for {
              N: 1 -> [_]
              tunnel: w367 -> [w373]
              shift-right: [w375] -> w370
              shift-left: w369 -> [w374]
              tunnel: w366 -> [w371]
              i -> [w372]
              n97 = property on="I slider 17" class="Slide (strict)"(error in=w374, "Active Slider"=w372, "Slider Colors"=w373, "HousingColor"=w371) -> (error out=w375:errorcluster)  [unwired: 1 in, 1 out]
            }
          }
          frame 18 {
            n98 = for {
              N: 1 -> [_]
              shift-right: [w385] -> w380
              shift-left: w379 -> [w384]
              tunnel: w377 -> [w382]
              tunnel: w376 -> [w381]
              i -> [w383]
              n99 = property on="I slider 18" class="Slide (strict)"(error in=w384, "Active Slider"=w383, "Slider Colors"=w382, "HousingColor"=w381) -> (error out=w385:errorcluster)  [unwired: 1 in, 1 out]
            }
          }
          frame 19 {
            n100 = for {
              N: 1 -> [_]
              tunnel: w387 -> [w393]
              shift-right: [w395] -> w390
              shift-left: w389 -> [w394]
              tunnel: w386 -> [w391]
              i -> [w392]
              n101 = property on="I slider 19" class="Slide (strict)"(error in=w394, "Active Slider"=w392, "Slider Colors"=w393, "HousingColor"=w391) -> (error out=w395:errorcluster)  [unwired: 1 in, 1 out]
            }
          }
          frame 20 {
            n102 = for {
              N: 1 -> [_]
              tunnel: w397 -> [w403]
              shift-right: [w405] -> w400
              shift-left: w399 -> [w404]
              tunnel: w396 -> [w401]
              i -> [w402]
              n103 = property on="I slider 20" class="Slide (strict)"(error in=w404, "Active Slider"=w402, "Slider Colors"=w403, "HousingColor"=w401) -> (error out=w405:errorcluster)  [unwired: 1 in, 1 out]
            }
          }
          frame 26, Default {
          }
        }
      }
      n104 = disable-structure shown="Disabled" {
        frame Disabled {
          n105 = case shown="13" {
            selector: _ -> [_ _ _ _ _ _ _ _ _ _ _ _ _ _ _ _ _ _ _ _ _ _]
            tunnel: _ -> [w30 w37 w42 w54 w62 w70 w78 w86 w94 w102 w110 w118 w126 w134 w142 w150 w158 w166 w174 w182 w190 w192]
            tunnel: [w27 w35 w41 w48 w56 w64 w72 w80 w88 w96 w104 w112 w120 w128 w136 w144 w152 w160 w168 w176 w184 w192] -> _
            tunnel: _ -> [w28 w31 _ w50 w58 w66 w74 w82 w90 w98 w106 w114 w122 w130 w138 w146 w154 w162 w170 w178 w186 _]
            tunnel: _ -> [w25 w33 w40 _ _ _ _ _ _ _ _ _ _ _ _ _ _ _ _ _ _ _]
            tunnel: _ -> [w24 w32 w39 _ _ _ _ _ _ _ _ _ _ _ _ _ _ _ _ _ _ _]
            frame 0 {
              n106 = Unbundle By Name(w28) -> ("Imaximum"=w26)
              n107 = property on="Property Node" class="Slide (strict)"(error in=w30, "Slider Colors"=w24, "Minimum"=0.0 ("Data Entry Limits:Minimum"), "Maximum"=w26, "HousingColor"=w25) -> (error out=w27:errorcluster)  [unwired: 1 in, 1 out]
            }
            frame 1 {
              n108 = Unbundle By Name(w31) -> ("Imaximum"=w34)
              n109 = property on="Property Node" class="Slide (strict)"(error in=w37, "Slider Colors"=w32, "Minimum"=0.0 ("Data Entry Limits:Minimum"), "Maximum"=w34, "HousingColor"=w33) -> (error out=w35:errorcluster)  [unwired: 1 in, 1 out]
            }
            frame 2 {
              n110 = for {
                N: 3 -> [_]
                tunnel: w40 -> [w45]
                tunnel: w39 -> [w44]
                shift-right: [w46] -> w41
                shift-left: w42 -> [w47]
                i -> [w43]
                n111 = property on="Property Node" class="Slide (strict)"(error in=w47, "Active Slider"=w43, "Slider Colors"=w44, "HousingColor"=w45) -> (error out=w46:errorcluster)  [unwired: 1 in, 1 out]
              }
            }
            frame 3 {
              n112 = Unbundle By Name(w50) -> ("Imaximum"=w49)
              n113 = property on="Property Node" class="Slide (strict)"(error in=w54, "BG Color"=16185337.0 ("Plot Area:Colors:BG Color"), "FGColor"=u32 0 ("Plot Area:Colors:FG Color"), "Minimum"=-10.0 ("Data Entry Limits:Minimum"), "Maximum"=w49, "BGColor"=u32 100 ("Housing Colors:BG Color")) -> (error out=w48:errorcluster)  [unwired: 1 in, 1 out]
            }
            frame 4 {
              n114 = Unbundle By Name(w58) -> ("Imaximum"=w57)
              n115 = property on="Property Node" class="Slide (strict)"(error in=w62, "BG Color"=16185337.0 ("Plot Area:Colors:BG Color"), "FGColor"=u32 0 ("Plot Area:Colors:FG Color"), "Minimum"=-10.0 ("Data Entry Limits:Minimum"), "Maximum"=w57, "BGColor"=u32 100 ("Housing Colors:BG Color")) -> (error out=w56:errorcluster)  [unwired: 1 in, 1 out]
            }
            frame 5 {
              n116 = Unbundle By Name(w66) -> ("Imaximum"=w65)
              n117 = property on="Property Node" class="Slide (strict)"(error in=w70, "BG Color"=16185337.0 ("Plot Area:Colors:BG Color"), "FGColor"=u32 0 ("Plot Area:Colors:FG Color"), "Minimum"=-10.0 ("Data Entry Limits:Minimum"), "Maximum"=w65, "BGColor"=u32 100 ("Housing Colors:BG Color")) -> (error out=w64:errorcluster)  [unwired: 1 in, 1 out]
            }
            frame 6 {
              n118 = Unbundle By Name(w74) -> ("Imaximum"=w73)
              n119 = property on="Property Node" class="Slide (strict)"(error in=w78, "BG Color"=16185337.0 ("Plot Area:Colors:BG Color"), "FGColor"=u32 0 ("Plot Area:Colors:FG Color"), "Minimum"=-10.0 ("Data Entry Limits:Minimum"), "Maximum"=w73, "BGColor"=u32 100 ("Housing Colors:BG Color")) -> (error out=w72:errorcluster)  [unwired: 1 in, 1 out]
            }
            frame 7 {
              n120 = Unbundle By Name(w82) -> ("Imaximum"=w81)
              n121 = property on="Property Node" class="Slide (strict)"(error in=w86, "BG Color"=16185337.0 ("Plot Area:Colors:BG Color"), "FGColor"=u32 0 ("Plot Area:Colors:FG Color"), "Minimum"=-10.0 ("Data Entry Limits:Minimum"), "Maximum"=w81, "BGColor"=u32 100 ("Housing Colors:BG Color")) -> (error out=w80:errorcluster)  [unwired: 1 in, 1 out]
            }
            frame 8 {
              n122 = Unbundle By Name(w90) -> ("Imaximum"=w89)
              n123 = property on="Property Node" class="Slide (strict)"(error in=w94, "BG Color"=16185337.0 ("Plot Area:Colors:BG Color"), "FGColor"=u32 0 ("Plot Area:Colors:FG Color"), "Minimum"=-10.0 ("Data Entry Limits:Minimum"), "Maximum"=w89, "BGColor"=u32 100 ("Housing Colors:BG Color")) -> (error out=w88:errorcluster)  [unwired: 1 in, 1 out]
            }
            frame 9 {
              n124 = Unbundle By Name(w98) -> ("Imaximum"=w97)
              n125 = property on="Property Node" class="Slide (strict)"(error in=w102, "BG Color"=16185337.0 ("Plot Area:Colors:BG Color"), "FGColor"=u32 0 ("Plot Area:Colors:FG Color"), "Minimum"=-10.0 ("Data Entry Limits:Minimum"), "Maximum"=w97, "BGColor"=u32 100 ("Housing Colors:BG Color")) -> (error out=w96:errorcluster)  [unwired: 1 in, 1 out]
            }
            frame 10 {
              n126 = Unbundle By Name(w106) -> ("Imaximum"=w105)
              n127 = property on="Property Node" class="Slide (strict)"(error in=w110, "BG Color"=16185337.0 ("Plot Area:Colors:BG Color"), "FGColor"=u32 0 ("Plot Area:Colors:FG Color"), "Minimum"=-10.0 ("Data Entry Limits:Minimum"), "Maximum"=w105, "BGColor"=u32 100 ("Housing Colors:BG Color")) -> (error out=w104:errorcluster)  [unwired: 1 in, 1 out]
            }
            frame 11 {
              n128 = Unbundle By Name(w114) -> ("Imaximum"=w113)
              n129 = property on="Property Node" class="Slide (strict)"(error in=w118, "BG Color"=16185337.0 ("Plot Area:Colors:BG Color"), "FGColor"=u32 0 ("Plot Area:Colors:FG Color"), "Minimum"=-10.0 ("Data Entry Limits:Minimum"), "Maximum"=w113, "BGColor"=u32 100 ("Housing Colors:BG Color")) -> (error out=w112:errorcluster)  [unwired: 1 in, 1 out]
            }
            frame 12 {
              n130 = Unbundle By Name(w122) -> ("Imaximum"=w121)
              n131 = property on="Property Node" class="Slide (strict)"(error in=w126, "BG Color"=16185337.0 ("Plot Area:Colors:BG Color"), "FGColor"=u32 0 ("Plot Area:Colors:FG Color"), "Minimum"=-10.0 ("Data Entry Limits:Minimum"), "Maximum"=w121, "BGColor"=u32 100 ("Housing Colors:BG Color")) -> (error out=w120:errorcluster)  [unwired: 1 in, 1 out]
            }
            frame 13 {
              n132 = Unbundle By Name(w130) -> ("Imaximum"=w129)
              n133 = property on="Property Node" class="Slide (strict)"(error in=w134, "BG Color"=16185337.0 ("Plot Area:Colors:BG Color"), "FGColor"=u32 0 ("Plot Area:Colors:FG Color"), "Minimum"=-10.0 ("Data Entry Limits:Minimum"), "Maximum"=w129, "BGColor"=u32 100 ("Housing Colors:BG Color")) -> (error out=w128:errorcluster)  [unwired: 1 in, 1 out]
            }
            frame 14 {
              n134 = Unbundle By Name(w138) -> ("Imaximum"=w137)
              n135 = property on="Property Node" class="Slide (strict)"(error in=w142, "BG Color"=16185337.0 ("Plot Area:Colors:BG Color"), "FGColor"=u32 0 ("Plot Area:Colors:FG Color"), "Minimum"=-10.0 ("Data Entry Limits:Minimum"), "Maximum"=w137, "BGColor"=u32 100 ("Housing Colors:BG Color")) -> (error out=w136:errorcluster)  [unwired: 1 in, 1 out]
            }
            frame 15 {
              n136 = Unbundle By Name(w146) -> ("Imaximum"=w145)
              n137 = property on="Property Node" class="Slide (strict)"(error in=w150, "BG Color"=16185337.0 ("Plot Area:Colors:BG Color"), "FGColor"=u32 0 ("Plot Area:Colors:FG Color"), "Minimum"=-10.0 ("Data Entry Limits:Minimum"), "Maximum"=w145, "BGColor"=u32 100 ("Housing Colors:BG Color")) -> (error out=w144:errorcluster)  [unwired: 1 in, 1 out]
            }
            frame 16 {
              n138 = Unbundle By Name(w154) -> ("Imaximum"=w153)
              n139 = property on="Property Node" class="Slide (strict)"(error in=w158, "BG Color"=16185337.0 ("Plot Area:Colors:BG Color"), "FGColor"=u32 0 ("Plot Area:Colors:FG Color"), "Minimum"=-10.0 ("Data Entry Limits:Minimum"), "Maximum"=w153, "BGColor"=u32 100 ("Housing Colors:BG Color")) -> (error out=w152:errorcluster)  [unwired: 1 in, 1 out]
            }
            frame 17 {
              n140 = Unbundle By Name(w162) -> ("Imaximum"=w161)
              n141 = property on="Property Node" class="Slide (strict)"(error in=w166, "BG Color"=16185337.0 ("Plot Area:Colors:BG Color"), "FGColor"=u32 0 ("Plot Area:Colors:FG Color"), "Minimum"=-10.0 ("Data Entry Limits:Minimum"), "Maximum"=w161, "BGColor"=u32 100 ("Housing Colors:BG Color")) -> (error out=w160:errorcluster)  [unwired: 1 in, 1 out]
            }
            frame 18 {
              n142 = Unbundle By Name(w170) -> ("Imaximum"=w169)
              n143 = property on="Property Node" class="Slide (strict)"(error in=w174, "BG Color"=16185337.0 ("Plot Area:Colors:BG Color"), "FGColor"=u32 0 ("Plot Area:Colors:FG Color"), "Minimum"=-10.0 ("Data Entry Limits:Minimum"), "Maximum"=w169, "BGColor"=u32 100 ("Housing Colors:BG Color")) -> (error out=w168:errorcluster)  [unwired: 1 in, 1 out]
            }
            frame 19 {
              n144 = Unbundle By Name(w178) -> ("Imaximum"=w177)
              n145 = property on="Property Node" class="Slide (strict)"(error in=w182, "BG Color"=16185337.0 ("Plot Area:Colors:BG Color"), "FGColor"=u32 0 ("Plot Area:Colors:FG Color"), "Minimum"=-10.0 ("Data Entry Limits:Minimum"), "Maximum"=w177, "BGColor"=u32 100 ("Housing Colors:BG Color")) -> (error out=w176:errorcluster)  [unwired: 1 in, 1 out]
            }
            frame 20 {
              n146 = Unbundle By Name(w186) -> ("Imaximum"=w185)
              n147 = property on="Property Node" class="Slide (strict)"(error in=w190, "BG Color"=16185337.0 ("Plot Area:Colors:BG Color"), "FGColor"=u32 0 ("Plot Area:Colors:FG Color"), "Minimum"=-10.0 ("Data Entry Limits:Minimum"), "Maximum"=w185, "BGColor"=u32 100 ("Housing Colors:BG Color")) -> (error out=w184:errorcluster)  [unwired: 1 in, 1 out]
            }
            frame 21, Default {
            }
          }
        }
        frame Enabled {
        }
      }
      n148 = Merge Errors(w22, w21) -> (w20:errorcluster)
    }
    frame #1 {
      # "Plot"
      n149 = while {
        tunnel: w679 -> [w702]
        shift-right: [w696] -> w669
        shift-left: w670 -> [w701]
        tunnel: [w700] -> w666
        tunnel: w678 -> [w699]
        tunnel: [w698] -> w677
        tunnel: w676 -> [w693]
        stop <- w692 stop-if-true
        # "Remark: timeout limits execution speed\nin case an error occurs"
        n150 = Wait on Notification(notifier=w702, timeout in ms (-1)=w693, error in (no error)=w701) -> (notifier out=w700:refnum<notifier>, notification=w691:T3, timed out?=w695:bool, error out=w697:errorcluster)  [unwired: 1 in]
        n151 = case shown="False" w695 {
          tunnel: w691 -> [_ _]
          tunnel: w691 -> [w707 _]
          tunnel: w691 -> [w704 _]
          frame False {
            n152 = Unbundle By Name(w707) -> ("Lines"=w706:T5)
            n153 = Unbundle By Name(w704) -> ("Buses"=w703:T6)
            n154 = Array Size(array=w706) -> (size(s)=w705:i32)
            n155 = for {
              tunnel: w703 -> [w925] mode=indexing
              tunnel: w703 -> [w920]
              i -> [w924]
              n156 = Unbundle By Name(w925) -> ("Iinjected"=w923:cdb[], "Sinjected"=w922:cdb[])
              n157 = case shown="True" TRUE {
                tunnel: w924 -> [_ w929]
                tunnel: w922 -> [_ w928]
                tunnel: w923 -> [_ w927]
                tunnel: w920 -> [_ w926]
                frame False {
                }
                frame True {
                  n158 = case shown="14" w929 {
                    tunnel: w927 -> [_ w948 w963 w982 w997 w1016 w1031 w1046 w1061 w1067 w1098 w1103 w1135 w1136 w1172 w1191 w1210 w1229 w1248 w1251 w1263 w1275 w1287 w1299 w1311 w1322 w1333]
                    tunnel: w928 -> [_ w947 w962 w981 w996 w1015 w1030 w1045 w1060 w1066 w1097 w1104 w1134 w1137 w1171 w1190 w1209 w1228 w1247 w1253 w1265 w1277 w1289 w1301 w1313 w1324 w1335]
                    tunnel: w926 -> [_ _ _ _ _ _ _ _ _ w1068 _ w1105 _ w1140 _ _ _ _ _ _ _ _ _ _ _ _ _]
                    frame 100, Default {
                    }
                    frame 0 {
                      w930 = 1000.0 ("y")
                      n159 = Complex To Re/Im(x + iy=w947) -> (x=w946:dbl[], y=w945:dbl[])
                      n160 = Absolute Value(x=w948) -> (abs(x)=w944:dbl[])
                      n161 = Add Array Elements(numeric array=w944) -> (sum=w943:dbl)
                      n162 = Add Array Elements(numeric array=w946) -> (sum=w937:dbl)
                      n163 = Add Array Elements(numeric array=w945) -> (sum=w939:dbl)
                      n164 = Divide(x=w943, y=3.0) -> (x/y=w931:dbl)
                      n165 = Round To Nearest(number=w937) -> (nearest integer value=w936:dbl)
                      n166 = Round To Nearest(number=w939) -> (nearest integer value=w938:dbl)
                      n167 = Multiply(x=w931, y=w930) -> (x*y=w932:dbl)
                      n168 = Round To Nearest(number=w932) -> (nearest integer value=w933:dbl)
                      n169 = Divide(x=w936, y=w930) -> (x/y=→"kW":dbl)
                      n170 = Divide(x=w938, y=w930) -> (x/y=→"?VkVAr":dbl)
                      n171 = Divide(x=w933, y=w930) -> (x/y=w934:dbl)
                      n172 = node(w934) -> (→"A":dbl[unit])
                    }
                    frame 1 {
                      w949 = 1000.0 ("y")
                      n173 = Complex To Re/Im(x + iy=w962) -> (x=w961:dbl[], y=w960:dbl[])
                      n174 = Absolute Value(x=w963) -> (abs(x)=w959:dbl[])
                      n175 = Add Array Elements(numeric array=w959) -> (sum=w958:dbl)
                      n176 = Add Array Elements(numeric array=w961) -> (sum=w954:dbl)
                      n177 = Add Array Elements(numeric array=w960) -> (sum=w956:dbl)
                      n178 = Divide(x=w958, y=3.0) -> (x/y=w950:dbl)
                      n179 = Round To Nearest(number=w954) -> (nearest integer value=w953:dbl)
                      n180 = Round To Nearest(number=w956) -> (nearest integer value=w955:dbl)
                      n181 = Multiply(x=w950, y=w949) -> (x*y=w951:dbl)
                      n182 = Round To Nearest(number=w951) -> (nearest integer value=w952:dbl)
                      n183 = Divide(x=w953, y=w949) -> ()  [unwired: 1 out]
                      n184 = Divide(x=w955, y=w949) -> ()  [unwired: 1 out]
                      n185 = Divide(x=w952, y=w949) -> ()  [unwired: 1 out]
                    }
                    frame 2 {
                      w968 = 1000.0 ("y")
                      n186 = Complex To Re/Im(x + iy=w981) -> (x=w980:dbl[], y=w979:dbl[])
                      n187 = Absolute Value(x=w982) -> (abs(x)=w978:dbl[])
                      n188 = Add Array Elements(numeric array=w978) -> (sum=w977:dbl)
                      n189 = Add Array Elements(numeric array=w980) -> (sum=w973:dbl)
                      n190 = Add Array Elements(numeric array=w979) -> (sum=w975:dbl)
                      n191 = Divide(x=w977, y=3.0) -> (x/y=w969:dbl)
                      n192 = Round To Nearest(number=w973) -> (nearest integer value=w972:dbl)
                      n193 = Round To Nearest(number=w975) -> (nearest integer value=w974:dbl)
                      n194 = Multiply(x=w969, y=w968) -> (x*y=w970:dbl)
                      n195 = Round To Nearest(number=w970) -> (nearest integer value=w971:dbl)
                      n196 = Divide(x=w972, y=w968) -> (x/y=→"kW":dbl)
                      n197 = Divide(x=w974, y=w968) -> (x/y=→"?VkVAr":dbl)
                      n198 = Divide(x=w971, y=w968) -> (x/y=w964:dbl)
                      n199 = node(w964) -> (→"A":dbl[unit])
                    }
                    frame 3 {
                      w983 = 1000.0 ("y")
                      n200 = Complex To Re/Im(x + iy=w996) -> (x=w995:dbl[], y=w994:dbl[])
                      n201 = Absolute Value(x=w997) -> (abs(x)=w993:dbl[])
                      n202 = Add Array Elements(numeric array=w993) -> (sum=w992:dbl)
                      n203 = Add Array Elements(numeric array=w995) -> (sum=w988:dbl)
                      n204 = Add Array Elements(numeric array=w994) -> (sum=w990:dbl)
                      n205 = Divide(x=w992, y=3.0) -> (x/y=w984:dbl)
                      n206 = Round To Nearest(number=w988) -> (nearest integer value=w987:dbl)
                      n207 = Round To Nearest(number=w990) -> (nearest integer value=w989:dbl)
                      n208 = Multiply(x=w984, y=w983) -> (x*y=w985:dbl)
                      n209 = Round To Nearest(number=w985) -> (nearest integer value=w986:dbl)
                      n210 = Divide(x=w987, y=w983) -> ()  [unwired: 1 out]
                      n211 = Divide(x=w989, y=w983) -> ()  [unwired: 1 out]
                      n212 = Divide(x=w986, y=w983) -> ()  [unwired: 1 out]
                    }
                    frame 4 {
                      w998 = 1000.0 ("y")
                      n213 = Complex To Re/Im(x + iy=w1015) -> (x=w1014:dbl[], y=w1013:dbl[])
                      n214 = Absolute Value(x=w1016) -> (abs(x)=w1012:dbl[])
                      n215 = Add Array Elements(numeric array=w1012) -> (sum=w1011:dbl)
                      n216 = Add Array Elements(numeric array=w1014) -> (sum=w1005:dbl)
                      n217 = Add Array Elements(numeric array=w1013) -> (sum=w1007:dbl)
                      n218 = Divide(x=w1011, y=3.0) -> (x/y=w999:dbl)
                      n219 = Round To Nearest(number=w1005) -> (nearest integer value=w1004:dbl)
                      n220 = Round To Nearest(number=w1007) -> (nearest integer value=w1006:dbl)
                      n221 = Multiply(x=w999, y=w998) -> (x*y=w1000:dbl)
                      n222 = Round To Nearest(number=w1000) -> (nearest integer value=w1001:dbl)
                      n223 = Divide(x=w1004, y=w998) -> (x/y=→"kW":dbl)
                      n224 = Divide(x=w1006, y=w998) -> (x/y=→"?VkVAr":dbl)
                      n225 = Divide(x=w1001, y=w998) -> (x/y=w1002:dbl)
                      n226 = node(w1002) -> (→"A":dbl[unit])
                    }
                    frame 5 {
                      w1017 = 1000.0 ("y")
                      n227 = Complex To Re/Im(x + iy=w1030) -> (x=w1029:dbl[], y=w1028:dbl[])
                      n228 = Absolute Value(x=w1031) -> (abs(x)=w1027:dbl[])
                      n229 = Add Array Elements(numeric array=w1027) -> (sum=w1026:dbl)
                      n230 = Add Array Elements(numeric array=w1029) -> (sum=w1022:dbl)
                      n231 = Add Array Elements(numeric array=w1028) -> (sum=w1024:dbl)
                      n232 = Divide(x=w1026, y=3.0) -> (x/y=w1018:dbl)
                      n233 = Round To Nearest(number=w1022) -> (nearest integer value=w1021:dbl)
                      n234 = Round To Nearest(number=w1024) -> (nearest integer value=w1023:dbl)
                      n235 = Multiply(x=w1018, y=w1017) -> (x*y=w1019:dbl)
                      n236 = Round To Nearest(number=w1019) -> (nearest integer value=w1020:dbl)
                      n237 = Divide(x=w1021, y=w1017) -> ()  [unwired: 1 out]
                      n238 = Divide(x=w1023, y=w1017) -> ()  [unwired: 1 out]
                      n239 = Divide(x=w1020, y=w1017) -> ()  [unwired: 1 out]
                    }
                    frame 6 {
                      w1032 = 1000.0 ("y")
                      n240 = Complex To Re/Im(x + iy=w1045) -> (x=w1044:dbl[], y=w1043:dbl[])
                      n241 = Absolute Value(x=w1046) -> (abs(x)=w1042:dbl[])
                      n242 = Add Array Elements(numeric array=w1042) -> (sum=w1041:dbl)
                      n243 = Add Array Elements(numeric array=w1044) -> (sum=w1037:dbl)
                      n244 = Add Array Elements(numeric array=w1043) -> (sum=w1039:dbl)
                      n245 = Divide(x=w1041, y=3.0) -> (x/y=w1033:dbl)
                      n246 = Round To Nearest(number=w1037) -> (nearest integer value=w1036:dbl)
                      n247 = Round To Nearest(number=w1039) -> (nearest integer value=w1038:dbl)
                      n248 = Multiply(x=w1033, y=w1032) -> (x*y=w1034:dbl)
                      n249 = Round To Nearest(number=w1034) -> (nearest integer value=w1035:dbl)
                      n250 = Divide(x=w1036, y=w1032) -> ()  [unwired: 1 out]
                      n251 = Divide(x=w1038, y=w1032) -> ()  [unwired: 1 out]
                      n252 = Divide(x=w1035, y=w1032) -> ()  [unwired: 1 out]
                    }
                    frame 7 {
                      w1047 = 1000.0 ("y")
                      n253 = Complex To Re/Im(x + iy=w1060) -> (x=w1059:dbl[], y=w1058:dbl[])
                      n254 = Absolute Value(x=w1061) -> (abs(x)=w1057:dbl[])
                      n255 = Add Array Elements(numeric array=w1057) -> (sum=w1056:dbl)
                      n256 = Add Array Elements(numeric array=w1059) -> (sum=w1052:dbl)
                      n257 = Add Array Elements(numeric array=w1058) -> (sum=w1054:dbl)
                      n258 = Divide(x=w1056, y=3.0) -> (x/y=w1048:dbl)
                      n259 = Round To Nearest(number=w1052) -> (nearest integer value=w1051:dbl)
                      n260 = Round To Nearest(number=w1054) -> (nearest integer value=w1053:dbl)
                      n261 = Multiply(x=w1048, y=w1047) -> (x*y=w1049:dbl)
                      n262 = Round To Nearest(number=w1049) -> (nearest integer value=w1050:dbl)
                      n263 = Divide(x=w1051, y=w1047) -> ()  [unwired: 1 out]
                      n264 = Divide(x=w1053, y=w1047) -> ()  [unwired: 1 out]
                      n265 = Divide(x=w1050, y=w1047) -> ()  [unwired: 1 out]
                    }
                    frame 8 {
                      w1071 = 1000.0 ("y")
                      n266 = Index Array(array=w1068, index=16) -> (element=w1069:T7)
                      n267 = Unbundle By Name(w1069) -> ()  [unwired: 2 out]
                      n268 = Complex To Re/Im(x + iy=w1066) -> (x=w1083:dbl[], y=w1082:dbl[])
                      n269 = Absolute Value(x=w1067) -> (abs(x)=w1081:dbl[])
                      n270 = Add Array Elements(numeric array=w1081) -> (sum=w1080:dbl)
                      n271 = Add Array Elements(numeric array=w1083) -> (sum=w1076:dbl)
                      n272 = Add Array Elements(numeric array=w1082) -> (sum=w1078:dbl)
                      n273 = Divide(x=w1080, y=3.0) -> (x/y=w1072:dbl)
                      n274 = Round To Nearest(number=w1076) -> (nearest integer value=w1075:dbl)
                      n275 = Round To Nearest(number=w1078) -> (nearest integer value=w1077:dbl)
                      n276 = Multiply(x=w1072, y=w1071) -> (x*y=w1073:dbl)
                      n277 = Round To Nearest(number=w1073) -> (nearest integer value=w1074:dbl)
                      n278 = Divide(x=w1075, y=w1071) -> (x/y=→"kW":dbl)
                      n279 = Divide(x=w1077, y=w1071) -> (x/y=→"?VkVAr":dbl)
                      n280 = Divide(x=w1074, y=w1071) -> (x/y=w1062:dbl)
                      n281 = node(w1062) -> (→"A":dbl[unit])
                    }
                    frame 9 {
                      w1084 = 1000.0 ("y")
                      n282 = Complex To Re/Im(x + iy=w1097) -> (x=w1096:dbl[], y=w1095:dbl[])
                      n283 = Absolute Value(x=w1098) -> (abs(x)=w1094:dbl[])
                      n284 = Add Array Elements(numeric array=w1094) -> (sum=w1093:dbl)
                      n285 = Add Array Elements(numeric array=w1096) -> (sum=w1089:dbl)
                      n286 = Add Array Elements(numeric array=w1095) -> (sum=w1091:dbl)
                      n287 = Divide(x=w1093, y=3.0) -> (x/y=w1085:dbl)
                      n288 = Round To Nearest(number=w1089) -> (nearest integer value=w1088:dbl)
                      n289 = Round To Nearest(number=w1091) -> (nearest integer value=w1090:dbl)
                      n290 = Multiply(x=w1085, y=w1084) -> (x*y=w1086:dbl)
                      n291 = Round To Nearest(number=w1086) -> (nearest integer value=w1087:dbl)
                      n292 = Divide(x=w1088, y=w1084) -> ()  [unwired: 1 out]
                      n293 = Divide(x=w1090, y=w1084) -> ()  [unwired: 1 out]
                      n294 = Divide(x=w1087, y=w1084) -> ()  [unwired: 1 out]
                    }
                    frame 10 {
                      w1108 = 1000.0 ("y")
                      n295 = Index Array(array=w1105, index=15) -> (element=w1106:T7)
                      n296 = Unbundle By Name(w1106) -> ()  [unwired: 2 out]
                      n297 = Complex To Re/Im(x + iy=w1104) -> (x=w1120:dbl[], y=w1119:dbl[])
                      n298 = Absolute Value(x=w1103) -> (abs(x)=w1118:dbl[])
                      n299 = Add Array Elements(numeric array=w1118) -> (sum=w1117:dbl)
                      n300 = Add Array Elements(numeric array=w1120) -> (sum=w1113:dbl)
                      n301 = Add Array Elements(numeric array=w1119) -> (sum=w1115:dbl)
                      n302 = Divide(x=w1117, y=3.0) -> (x/y=w1109:dbl)
                      n303 = Round To Nearest(number=w1113) -> (nearest integer value=w1112:dbl)
                      n304 = Round To Nearest(number=w1115) -> (nearest integer value=w1114:dbl)
                      n305 = Multiply(x=w1109, y=w1108) -> (x*y=w1110:dbl)
                      n306 = Round To Nearest(number=w1110) -> (nearest integer value=w1111:dbl)
                      n307 = Divide(x=w1112, y=w1108) -> (x/y=→"kW":dbl)
                      n308 = Divide(x=w1114, y=w1108) -> (x/y=→"?VkVAr":dbl)
                      n309 = Divide(x=w1111, y=w1108) -> (x/y=w1099:dbl)
                      n310 = node(w1099) -> (→"A":dbl[unit])
                    }
                    frame 11 {
                      w1121 = 1000.0 ("y")
                      n311 = Complex To Re/Im(x + iy=w1134) -> (x=w1133:dbl[], y=w1132:dbl[])
                      n312 = Absolute Value(x=w1135) -> (abs(x)=w1131:dbl[])
                      n313 = Add Array Elements(numeric array=w1131) -> (sum=w1130:dbl)
                      n314 = Add Array Elements(numeric array=w1133) -> (sum=w1126:dbl)
                      n315 = Add Array Elements(numeric array=w1132) -> (sum=w1128:dbl)
                      n316 = Divide(x=w1130, y=3.0) -> (x/y=w1122:dbl)
                      n317 = Round To Nearest(number=w1126) -> (nearest integer value=w1125:dbl)
                      n318 = Round To Nearest(number=w1128) -> (nearest integer value=w1127:dbl)
                      n319 = Multiply(x=w1122, y=w1121) -> (x*y=w1123:dbl)
                      n320 = Round To Nearest(number=w1123) -> (nearest integer value=w1124:dbl)
                      n321 = Divide(x=w1125, y=w1121) -> ()  [unwired: 1 out]
                      n322 = Divide(x=w1127, y=w1121) -> ()  [unwired: 1 out]
                      n323 = Divide(x=w1124, y=w1121) -> ()  [unwired: 1 out]
                    }
                    frame 12 {
                      w1141 = 1000.0 ("y")
                      n324 = Index Array(array=w1140, index=14) -> (element=w1138:T7)
                      n325 = Unbundle By Name(w1138) -> ()  [unwired: 2 out]
                      n326 = Complex To Re/Im(x + iy=w1137) -> (x=w1153:dbl[], y=w1152:dbl[])
                      n327 = Absolute Value(x=w1136) -> (abs(x)=w1151:dbl[])
                      n328 = Add Array Elements(numeric array=w1151) -> (sum=w1150:dbl)
                      n329 = Add Array Elements(numeric array=w1153) -> (sum=w1146:dbl)
                      n330 = Add Array Elements(numeric array=w1152) -> (sum=w1148:dbl)
                      n331 = Divide(x=w1150, y=3.0) -> (x/y=w1142:dbl)
                      n332 = Round To Nearest(number=w1146) -> (nearest integer value=w1145:dbl)
                      n333 = Round To Nearest(number=w1148) -> (nearest integer value=w1147:dbl)
                      n334 = Multiply(x=w1142, y=w1141) -> (x*y=w1143:dbl)
                      n335 = Round To Nearest(number=w1143) -> (nearest integer value=w1144:dbl)
                      n336 = Divide(x=w1145, y=w1141) -> ()  [unwired: 1 out]
                      n337 = Divide(x=w1147, y=w1141) -> ()  [unwired: 1 out]
                      n338 = Divide(x=w1144, y=w1141) -> ()  [unwired: 1 out]
                    }
                    frame 13 {
                      w1158 = 1000.0 ("y")
                      n339 = Complex To Re/Im(x + iy=w1171) -> (x=w1170:dbl[], y=w1169:dbl[])
                      n340 = Absolute Value(x=w1172) -> (abs(x)=w1168:dbl[])
                      n341 = Add Array Elements(numeric array=w1168) -> (sum=w1167:dbl)
                      n342 = Add Array Elements(numeric array=w1170) -> (sum=w1163:dbl)
                      n343 = Add Array Elements(numeric array=w1169) -> (sum=w1165:dbl)
                      n344 = Divide(x=w1167, y=3.0) -> (x/y=w1159:dbl)
                      n345 = Round To Nearest(number=w1163) -> (nearest integer value=w1162:dbl)
                      n346 = Round To Nearest(number=w1165) -> (nearest integer value=w1164:dbl)
                      n347 = Multiply(x=w1159, y=w1158) -> (x*y=w1160:dbl)
                      n348 = Round To Nearest(number=w1160) -> (nearest integer value=w1161:dbl)
                      n349 = Divide(x=w1162, y=w1158) -> (x/y=→"kW":dbl)
                      n350 = Divide(x=w1164, y=w1158) -> (x/y=→"?VkVAr":dbl)
                      n351 = Divide(x=w1161, y=w1158) -> (x/y=w1154:dbl)
                      n352 = node(w1154) -> (→"A":dbl[unit])
                    }
                    frame 14 {
                      w1177 = 1000.0 ("y")
                      n353 = Complex To Re/Im(x + iy=w1190) -> (x=w1189:dbl[], y=w1188:dbl[])
                      n354 = Absolute Value(x=w1191) -> (abs(x)=w1187:dbl[])
                      n355 = Add Array Elements(numeric array=w1187) -> (sum=w1186:dbl)
                      n356 = Add Array Elements(numeric array=w1189) -> (sum=w1182:dbl)
                      n357 = Add Array Elements(numeric array=w1188) -> (sum=w1184:dbl)
                      n358 = Divide(x=w1186, y=3.0) -> (x/y=w1178:dbl)
                      n359 = Round To Nearest(number=w1182) -> (nearest integer value=w1181:dbl)
                      n360 = Round To Nearest(number=w1184) -> (nearest integer value=w1183:dbl)
                      n361 = Multiply(x=w1178, y=w1177) -> (x*y=w1179:dbl)
                      n362 = Round To Nearest(number=w1179) -> (nearest integer value=w1180:dbl)
                      n363 = Divide(x=w1181, y=w1177) -> (x/y=→"kW":dbl)
                      n364 = Divide(x=w1183, y=w1177) -> (x/y=→"?VkVAr":dbl)
                      n365 = Divide(x=w1180, y=w1177) -> (x/y=w1173:dbl)
                      n366 = node(w1173) -> (→"A":dbl[unit])
                    }
                    frame 15 {
                      w1196 = 1000.0 ("y")
                      n367 = Complex To Re/Im(x + iy=w1209) -> (x=w1208:dbl[], y=w1207:dbl[])
                      n368 = Absolute Value(x=w1210) -> (abs(x)=w1206:dbl[])
                      n369 = Add Array Elements(numeric array=w1206) -> (sum=w1205:dbl)
                      n370 = Add Array Elements(numeric array=w1208) -> (sum=w1201:dbl)
                      n371 = Add Array Elements(numeric array=w1207) -> (sum=w1203:dbl)
                      n372 = Divide(x=w1205, y=3.0) -> (x/y=w1197:dbl)
                      n373 = Round To Nearest(number=w1201) -> (nearest integer value=w1200:dbl)
                      n374 = Round To Nearest(number=w1203) -> (nearest integer value=w1202:dbl)
                      n375 = Multiply(x=w1197, y=w1196) -> (x*y=w1198:dbl)
                      n376 = Round To Nearest(number=w1198) -> (nearest integer value=w1199:dbl)
                      n377 = Divide(x=w1200, y=w1196) -> (x/y=→"kW":dbl)
                      n378 = Divide(x=w1202, y=w1196) -> (x/y=→"?VkVAr":dbl)
                      n379 = Divide(x=w1199, y=w1196) -> (x/y=w1192:dbl)
                      n380 = node(w1192) -> (→"A":dbl[unit])
                    }
                    frame 16 {
                      w1215 = 1000.0 ("y")
                      n381 = Complex To Re/Im(x + iy=w1228) -> (x=w1227:dbl[], y=w1226:dbl[])
                      n382 = Absolute Value(x=w1229) -> (abs(x)=w1225:dbl[])
                      n383 = Add Array Elements(numeric array=w1225) -> (sum=w1224:dbl)
                      n384 = Add Array Elements(numeric array=w1227) -> (sum=w1220:dbl)
                      n385 = Add Array Elements(numeric array=w1226) -> (sum=w1222:dbl)
                      n386 = Divide(x=w1224, y=3.0) -> (x/y=w1216:dbl)
                      n387 = Round To Nearest(number=w1220) -> (nearest integer value=w1219:dbl)
                      n388 = Round To Nearest(number=w1222) -> (nearest integer value=w1221:dbl)
                      n389 = Multiply(x=w1216, y=w1215) -> (x*y=w1217:dbl)
                      n390 = Round To Nearest(number=w1217) -> (nearest integer value=w1218:dbl)
                      n391 = Divide(x=w1219, y=w1215) -> (x/y=→"kW":dbl)
                      n392 = Divide(x=w1221, y=w1215) -> (x/y=→"?VkVAr":dbl)
                      n393 = Divide(x=w1218, y=w1215) -> (x/y=w1211:dbl)
                      n394 = node(w1211) -> (→"A":dbl[unit])
                    }
                    frame 17 {
                      w1234 = 1000.0 ("y")
                      n395 = Complex To Re/Im(x + iy=w1247) -> (x=w1246:dbl[], y=w1245:dbl[])
                      n396 = Absolute Value(x=w1248) -> (abs(x)=w1244:dbl[])
                      n397 = Add Array Elements(numeric array=w1244) -> (sum=w1243:dbl)
                      n398 = Add Array Elements(numeric array=w1246) -> (sum=w1239:dbl)
                      n399 = Add Array Elements(numeric array=w1245) -> (sum=w1241:dbl)
                      n400 = Divide(x=w1243, y=3.0) -> (x/y=w1235:dbl)
                      n401 = Round To Nearest(number=w1239) -> (nearest integer value=w1238:dbl)
                      n402 = Round To Nearest(number=w1241) -> (nearest integer value=w1240:dbl)
                      n403 = Multiply(x=w1235, y=w1234) -> (x*y=w1236:dbl)
                      n404 = Round To Nearest(number=w1236) -> (nearest integer value=w1237:dbl)
                      n405 = Divide(x=w1238, y=w1234) -> (x/y=→"kW":dbl)
                      n406 = Divide(x=w1240, y=w1234) -> (x/y=→"?VkVAr":dbl)
                      n407 = Divide(x=w1237, y=w1234) -> (x/y=w1230:dbl)
                      n408 = node(w1230) -> (→"A":dbl[unit])
                    }
                    frame 18 {
                      w1256 = 1000.0 ("y")
                      n409 = Index Array(array=w1251) -> (element=w1250:cdb)  [unwired: 1 in]
                      n410 = Index Array(array=w1253) -> (element=w1252:cdb)  [unwired: 1 in]
                      n411 = Absolute Value(x=w1250) -> (abs(x)=w1255:dbl)
                      n412 = Absolute Value(x=w1252) -> (abs(x)=w1254:dbl)
                      n413 = Round To Nearest(number=w1254) -> (nearest integer value=w1260:dbl)
                      n414 = Multiply(x=w1255, y=w1256) -> (x*y=w1257:dbl)
                      n415 = Round To Nearest(number=w1257) -> (nearest integer value=w1258:dbl)
                      n416 = Divide(x=w1260, y=w1256) -> (x/y=→"kW":dbl)
                      n417 = Divide(x=w1258, y=w1256) -> (x/y=→"A":dbl)
                    }
                    frame 19 {
                      w1268 = 1000.0 ("y")
                      n418 = Index Array(array=w1263) -> (element=w1262:cdb)  [unwired: 1 in]
                      n419 = Index Array(array=w1265) -> (element=w1264:cdb)  [unwired: 1 in]
                      n420 = Absolute Value(x=w1262) -> (abs(x)=w1267:dbl)
                      n421 = Absolute Value(x=w1264) -> (abs(x)=w1266:dbl)
                      n422 = Round To Nearest(number=w1266) -> (nearest integer value=w1272:dbl)
                      n423 = Multiply(x=w1267, y=w1268) -> (x*y=w1269:dbl)
                      n424 = Round To Nearest(number=w1269) -> (nearest integer value=w1270:dbl)
                      n425 = Divide(x=w1272, y=w1268) -> (x/y=→"kW":dbl)
                      n426 = Divide(x=w1270, y=w1268) -> (x/y=→"A":dbl)
                    }
                    frame 20 {
                      w1280 = 1000.0 ("y")
                      n427 = Index Array(array=w1275) -> (element=w1274:cdb)  [unwired: 1 in]
                      n428 = Index Array(array=w1277) -> (element=w1276:cdb)  [unwired: 1 in]
                      n429 = Absolute Value(x=w1274) -> (abs(x)=w1279:dbl)
                      n430 = Absolute Value(x=w1276) -> (abs(x)=w1278:dbl)
                      n431 = Round To Nearest(number=w1278) -> (nearest integer value=w1284:dbl)
                      n432 = Multiply(x=w1279, y=w1280) -> (x*y=w1281:dbl)
                      n433 = Round To Nearest(number=w1281) -> (nearest integer value=w1282:dbl)
                      n434 = Divide(x=w1284, y=w1280) -> (x/y=→"kW":dbl)
                      n435 = Divide(x=w1282, y=w1280) -> (x/y=→"A":dbl)
                    }
                    frame 21 {
                      w1292 = 1000.0 ("y")
                      n436 = Index Array(array=w1287) -> (element=w1286:cdb)  [unwired: 1 in]
                      n437 = Index Array(array=w1289) -> (element=w1288:cdb)  [unwired: 1 in]
                      n438 = Absolute Value(x=w1286) -> (abs(x)=w1291:dbl)
                      n439 = Absolute Value(x=w1288) -> (abs(x)=w1290:dbl)
                      n440 = Round To Nearest(number=w1290) -> (nearest integer value=w1296:dbl)
                      n441 = Multiply(x=w1291, y=w1292) -> (x*y=w1293:dbl)
                      n442 = Round To Nearest(number=w1293) -> (nearest integer value=w1294:dbl)
                      n443 = Divide(x=w1296, y=w1292) -> (x/y=→"kW":dbl)
                      n444 = Divide(x=w1294, y=w1292) -> (x/y=→"A":dbl)
                    }
                    frame 22 {
                      w1304 = 1000.0 ("y")
                      n445 = Index Array(array=w1299) -> (element=w1298:cdb)  [unwired: 1 in]
                      n446 = Index Array(array=w1301) -> (element=w1300:cdb)  [unwired: 1 in]
                      n447 = Absolute Value(x=w1298) -> (abs(x)=w1303:dbl)
                      n448 = Absolute Value(x=w1300) -> (abs(x)=w1302:dbl)
                      n449 = Round To Nearest(number=w1302) -> (nearest integer value=w1308:dbl)
                      n450 = Multiply(x=w1303, y=w1304) -> (x*y=w1305:dbl)
                      n451 = Round To Nearest(number=w1305) -> (nearest integer value=w1306:dbl)
                      n452 = Divide(x=w1308, y=w1304) -> (x/y=→"kW":dbl)
                      n453 = Divide(x=w1306, y=w1304) -> (x/y=→"A":dbl)
                    }
                    frame 23 {
                      w1316 = 1000.0 ("y")
                      n454 = Index Array(array=w1311) -> (element=w1310:cdb)  [unwired: 1 in]
                      n455 = Index Array(array=w1313) -> (element=w1312:cdb)  [unwired: 1 in]
                      n456 = Absolute Value(x=w1310) -> (abs(x)=w1315:dbl)
                      n457 = Absolute Value(x=w1312) -> (abs(x)=w1314:dbl)
                      n458 = Round To Nearest(number=w1314) -> (nearest integer value=w1320:dbl)
                      n459 = Multiply(x=w1315, y=w1316) -> (x*y=w1317:dbl)
                      n460 = Round To Nearest(number=w1317) -> (nearest integer value=w1318:dbl)
                      n461 = Divide(x=w1320, y=w1316) -> (x/y=→"kW":dbl)
                      n462 = Divide(x=w1318, y=w1316) -> (x/y=→"A":dbl)
                    }
                    frame 25 {
                      w1327 = 1000.0 ("y")
                      n463 = Index Array(array=w1322) -> (element=w1321:cdb)  [unwired: 1 in]
                      n464 = Index Array(array=w1324) -> (element=w1323:cdb)  [unwired: 1 in]
                      n465 = Absolute Value(x=w1321) -> (abs(x)=w1326:dbl)
                      n466 = Absolute Value(x=w1323) -> (abs(x)=w1325:dbl)
                      n467 = Round To Nearest(number=w1325) -> (nearest integer value=w1330:dbl)
                      n468 = Multiply(x=w1326, y=w1327) -> (x*y=w1328:dbl)
                      n469 = Round To Nearest(number=w1328) -> (nearest integer value=w1329:dbl)
                      n470 = Divide(x=w1330, y=w1327) -> ()  [unwired: 1 out]
                      n471 = Divide(x=w1329, y=w1327) -> ()  [unwired: 1 out]
                    }
                    frame 24 {
                      w1338 = 1000.0 ("y")
                      n472 = Index Array(array=w1333) -> (element=w1332:cdb)  [unwired: 1 in]
                      n473 = Index Array(array=w1335) -> (element=w1334:cdb)  [unwired: 1 in]
                      n474 = Absolute Value(x=w1332) -> (abs(x)=w1337:dbl)
                      n475 = Absolute Value(x=w1334) -> (abs(x)=w1336:dbl)
                      n476 = Round To Nearest(number=w1336) -> (nearest integer value=w1342:dbl)
                      n477 = Multiply(x=w1337, y=w1338) -> (x*y=w1339:dbl)
                      n478 = Round To Nearest(number=w1339) -> (nearest integer value=w1340:dbl)
                      n479 = Divide(x=w1342, y=w1338) -> (x/y=→"kW":dbl)
                      n480 = Divide(x=w1340, y=w1338) -> (x/y=→"A":dbl)
                    }
                  }
                }
              }
            }
            n481 = for {
              N: w705 -> [_]
              tunnel: w706 -> [w1348] mode=indexing
              i -> [w1347]
              n482 = Unbundle By Name(w1348) -> ("Iforward"=w1345:cdb[], "Imaximum"=w1344:dbl)
              n483 = call "Plot Line Current.vi"("I_trip"=w1344, "I_line"=w1345) -> ("I-i"=w1346:T8)  [unwired: 1 in]
              n484 = case shown="True" TRUE {
                tunnel: w1347 -> [_ w1350]
                tunnel: w1346 -> [_ w1349]
                frame False {
                }
                frame True {
                  n485 = case shown="17" w1350 {
                    tunnel: w1349 -> [w1352 w1370 w1404 w1406 w1424 w1442 w1476 w1478 w1512 w1514 w1548 w1550 w1568 w1586 w1604 w1622 w1640 w1659 w1666 w1673 w1680 _]
                    frame 0 {
                      w1353 = 100.0 ("y")
                      n486 = Unbundle By Name(w1352) -> ("Phasor C"=w1365:dbl, "Phasor C"=w1359:dbl, "Phasor C"=w1357:dbl)
                      n487 = Absolute Value(x=w1365) -> (abs(x)=w1366:dbl)
                      n488 = Absolute Value(x=w1359) -> (abs(x)=w1358:dbl)
                      n489 = Absolute Value(x=w1357) -> (abs(x)=w1356:dbl)
                      n490 = Multiply(x=w1366, y=w1353) -> (x*y=w1367:dbl)
                      n491 = Multiply(x=w1358, y=w1353) -> (x*y=w1362:dbl)
                      n492 = Multiply(x=w1356, y=w1353) -> (x*y=w1360:dbl)
                      n493 = Round To Nearest(number=w1367) -> (nearest integer value=w1368:dbl)
                      n494 = Round To Nearest(number=w1362) -> (nearest integer value=w1363:dbl)
                      n495 = Round To Nearest(number=w1360) -> (nearest integer value=w1361:dbl)
                      n496 = Divide(x=w1368, y=w1353) -> (x/y=w1364:dbl)
                      n497 = Divide(x=w1363, y=w1353) -> (x/y=w1355:dbl)
                      n498 = Divide(x=w1361, y=w1353) -> (x/y=w1354:dbl)
                      n499 = Bundle(w1364, w1355, w1354) -> (→"I slider 0":cluster{dbl, dbl, dbl})  [unwired: 1 in]
                    }
                    frame 1 {
                      w1371 = 100.0 ("y")
                      n500 = Unbundle By Name(w1370) -> ("Phasor C"=w1383:dbl, "Phasor C"=w1377:dbl, "Phasor C"=w1375:dbl)
                      n501 = Absolute Value(x=w1383) -> (abs(x)=w1384:dbl)
                      n502 = Absolute Value(x=w1377) -> (abs(x)=w1376:dbl)
                      n503 = Absolute Value(x=w1375) -> (abs(x)=w1374:dbl)
                      n504 = Multiply(x=w1384, y=w1371) -> (x*y=w1385:dbl)
                      n505 = Multiply(x=w1376, y=w1371) -> (x*y=w1380:dbl)
                      n506 = Multiply(x=w1374, y=w1371) -> (x*y=w1378:dbl)
                      n507 = Round To Nearest(number=w1385) -> (nearest integer value=w1386:dbl)
                      n508 = Round To Nearest(number=w1380) -> (nearest integer value=w1381:dbl)
                      n509 = Round To Nearest(number=w1378) -> (nearest integer value=w1379:dbl)
                      n510 = Divide(x=w1386, y=w1371) -> (x/y=w1382:dbl)
                      n511 = Divide(x=w1381, y=w1371) -> (x/y=w1373:dbl)
                      n512 = Divide(x=w1379, y=w1371) -> (x/y=w1372:dbl)
                      n513 = Bundle(w1382, w1373, w1372) -> (→"I slider 1":cluster{dbl, dbl, dbl})  [unwired: 1 in]
                    }
                    frame 2 {
                      w1387 = 100.0 ("y")
                      n514 = Unbundle By Name(w1404) -> ("Phasor C"=w1399:dbl, "Phasor C"=w1393:dbl, "Phasor C"=w1391:dbl)
                      n515 = Absolute Value(x=w1399) -> (abs(x)=w1400:dbl)
                      n516 = Absolute Value(x=w1393) -> (abs(x)=w1392:dbl)
                      n517 = Absolute Value(x=w1391) -> (abs(x)=w1390:dbl)
                      n518 = Multiply(x=w1400, y=w1387) -> (x*y=w1401:dbl)
                      n519 = Multiply(x=w1392, y=w1387) -> (x*y=w1396:dbl)
                      n520 = Multiply(x=w1390, y=w1387) -> (x*y=w1394:dbl)
                      n521 = Round To Nearest(number=w1401) -> (nearest integer value=w1402:dbl)
                      n522 = Round To Nearest(number=w1396) -> (nearest integer value=w1397:dbl)
                      n523 = Round To Nearest(number=w1394) -> (nearest integer value=w1395:dbl)
                      n524 = Divide(x=w1402, y=w1387) -> (x/y=w1398:dbl)
                      n525 = Divide(x=w1397, y=w1387) -> (x/y=w1389:dbl)
                      n526 = Divide(x=w1395, y=w1387) -> (x/y=w1388:dbl)
                      n527 = Bundle(w1398, w1389, w1388) -> (→"I slider 2":cluster{dbl, dbl, dbl})  [unwired: 1 in]
                    }
                    frame 3 {
                      w1407 = 100.0 ("y")
                      n528 = Unbundle By Name(w1406) -> ("Phasor C"=w1419:dbl, "Phasor C"=w1413:dbl, "Phasor C"=w1411:dbl)
                      n529 = Absolute Value(x=w1419) -> (abs(x)=w1420:dbl)
                      n530 = Absolute Value(x=w1413) -> (abs(x)=w1412:dbl)
                      n531 = Absolute Value(x=w1411) -> (abs(x)=w1410:dbl)
                      n532 = Multiply(x=w1420, y=w1407) -> (x*y=w1421:dbl)
                      n533 = Multiply(x=w1412, y=w1407) -> (x*y=w1416:dbl)
                      n534 = Multiply(x=w1410, y=w1407) -> (x*y=w1414:dbl)
                      n535 = Round To Nearest(number=w1421) -> (nearest integer value=w1422:dbl)
                      n536 = Round To Nearest(number=w1416) -> (nearest integer value=w1417:dbl)
                      n537 = Round To Nearest(number=w1414) -> (nearest integer value=w1415:dbl)
                      n538 = Divide(x=w1422, y=w1407) -> (x/y=w1418:dbl)
                      n539 = Divide(x=w1417, y=w1407) -> (x/y=w1409:dbl)
                      n540 = Divide(x=w1415, y=w1407) -> (x/y=w1408:dbl)
                      n541 = Bundle(w1418, w1409, w1408) -> (→"I slider 3":cluster{dbl, dbl, dbl})  [unwired: 1 in]
                    }
                    frame 4 {
                      w1425 = 100.0 ("y")
                      n542 = Unbundle By Name(w1424) -> ("Phasor C"=w1437:dbl, "Phasor C"=w1431:dbl, "Phasor C"=w1429:dbl)
                      n543 = Absolute Value(x=w1437) -> (abs(x)=w1438:dbl)
                      n544 = Absolute Value(x=w1431) -> (abs(x)=w1430:dbl)
                      n545 = Absolute Value(x=w1429) -> (abs(x)=w1428:dbl)
                      n546 = Multiply(x=w1438, y=w1425) -> (x*y=w1439:dbl)
                      n547 = Multiply(x=w1430, y=w1425) -> (x*y=w1434:dbl)
                      n548 = Multiply(x=w1428, y=w1425) -> (x*y=w1432:dbl)
                      n549 = Round To Nearest(number=w1439) -> (nearest integer value=w1440:dbl)
                      n550 = Round To Nearest(number=w1434) -> (nearest integer value=w1435:dbl)
                      n551 = Round To Nearest(number=w1432) -> (nearest integer value=w1433:dbl)
                      n552 = Divide(x=w1440, y=w1425) -> (x/y=w1436:dbl)
                      n553 = Divide(x=w1435, y=w1425) -> (x/y=w1427:dbl)
                      n554 = Divide(x=w1433, y=w1425) -> (x/y=w1426:dbl)
                      n555 = Bundle(w1436, w1427, w1426) -> (→"I slider 4":cluster{dbl, dbl, dbl})  [unwired: 1 in]
                    }
                    frame 5 {
                      w1443 = 100.0 ("y")
                      n556 = Unbundle By Name(w1442) -> ("Phasor C"=w1455:dbl, "Phasor C"=w1449:dbl, "Phasor C"=w1447:dbl)
                      n557 = Absolute Value(x=w1455) -> (abs(x)=w1456:dbl)
                      n558 = Absolute Value(x=w1449) -> (abs(x)=w1448:dbl)
                      n559 = Absolute Value(x=w1447) -> (abs(x)=w1446:dbl)
                      n560 = Multiply(x=w1456, y=w1443) -> (x*y=w1457:dbl)
                      n561 = Multiply(x=w1448, y=w1443) -> (x*y=w1452:dbl)
                      n562 = Multiply(x=w1446, y=w1443) -> (x*y=w1450:dbl)
                      n563 = Round To Nearest(number=w1457) -> (nearest integer value=w1458:dbl)
                      n564 = Round To Nearest(number=w1452) -> (nearest integer value=w1453:dbl)
                      n565 = Round To Nearest(number=w1450) -> (nearest integer value=w1451:dbl)
                      n566 = Divide(x=w1458, y=w1443) -> (x/y=w1454:dbl)
                      n567 = Divide(x=w1453, y=w1443) -> (x/y=w1445:dbl)
                      n568 = Divide(x=w1451, y=w1443) -> (x/y=w1444:dbl)
                      n569 = Bundle(w1454, w1445, w1444) -> (→"I slider 5":cluster{dbl, dbl, dbl})  [unwired: 1 in]
                    }
                    frame 6 {
                      w1459 = 100.0 ("y")
                      n570 = Unbundle By Name(w1476) -> ("Phasor C"=w1471:dbl, "Phasor C"=w1465:dbl, "Phasor C"=w1463:dbl)
                      n571 = Absolute Value(x=w1471) -> (abs(x)=w1472:dbl)
                      n572 = Absolute Value(x=w1465) -> (abs(x)=w1464:dbl)
                      n573 = Absolute Value(x=w1463) -> (abs(x)=w1462:dbl)
                      n574 = Multiply(x=w1472, y=w1459) -> (x*y=w1473:dbl)
                      n575 = Multiply(x=w1464, y=w1459) -> (x*y=w1468:dbl)
                      n576 = Multiply(x=w1462, y=w1459) -> (x*y=w1466:dbl)
                      n577 = Round To Nearest(number=w1473) -> (nearest integer value=w1474:dbl)
                      n578 = Round To Nearest(number=w1468) -> (nearest integer value=w1469:dbl)
                      n579 = Round To Nearest(number=w1466) -> (nearest integer value=w1467:dbl)
                      n580 = Divide(x=w1474, y=w1459) -> (x/y=w1470:dbl)
                      n581 = Divide(x=w1469, y=w1459) -> (x/y=w1461:dbl)
                      n582 = Divide(x=w1467, y=w1459) -> (x/y=w1460:dbl)
                      n583 = Bundle(w1470, w1461, w1460) -> (→"I slider 6":cluster{dbl, dbl, dbl})  [unwired: 1 in]
                    }
                    frame 7 {
                      w1479 = 100.0 ("y")
                      n584 = Unbundle By Name(w1478) -> ("Phasor C"=w1491:dbl, "Phasor C"=w1485:dbl, "Phasor C"=w1483:dbl)
                      n585 = Absolute Value(x=w1491) -> (abs(x)=w1492:dbl)
                      n586 = Absolute Value(x=w1485) -> (abs(x)=w1484:dbl)
                      n587 = Absolute Value(x=w1483) -> (abs(x)=w1482:dbl)
                      n588 = Multiply(x=w1492, y=w1479) -> (x*y=w1493:dbl)
                      n589 = Multiply(x=w1484, y=w1479) -> (x*y=w1488:dbl)
                      n590 = Multiply(x=w1482, y=w1479) -> (x*y=w1486:dbl)
                      n591 = Round To Nearest(number=w1493) -> (nearest integer value=w1494:dbl)
                      n592 = Round To Nearest(number=w1488) -> (nearest integer value=w1489:dbl)
                      n593 = Round To Nearest(number=w1486) -> (nearest integer value=w1487:dbl)
                      n594 = Divide(x=w1494, y=w1479) -> (x/y=w1490:dbl)
                      n595 = Divide(x=w1489, y=w1479) -> (x/y=w1481:dbl)
                      n596 = Divide(x=w1487, y=w1479) -> (x/y=w1480:dbl)
                      n597 = Bundle(w1490, w1481, w1480) -> (→"I slider 7":cluster{dbl, dbl, dbl})  [unwired: 1 in]
                    }
                    frame 8 {
                      w1495 = 100.0 ("y")
                      n598 = Unbundle By Name(w1512) -> ("Phasor C"=w1507:dbl, "Phasor C"=w1501:dbl, "Phasor C"=w1499:dbl)
                      n599 = Absolute Value(x=w1507) -> (abs(x)=w1508:dbl)
                      n600 = Absolute Value(x=w1501) -> (abs(x)=w1500:dbl)
                      n601 = Absolute Value(x=w1499) -> (abs(x)=w1498:dbl)
                      n602 = Multiply(x=w1508, y=w1495) -> (x*y=w1509:dbl)
                      n603 = Multiply(x=w1500, y=w1495) -> (x*y=w1504:dbl)
                      n604 = Multiply(x=w1498, y=w1495) -> (x*y=w1502:dbl)
                      n605 = Round To Nearest(number=w1509) -> (nearest integer value=w1510:dbl)
                      n606 = Round To Nearest(number=w1504) -> (nearest integer value=w1505:dbl)
                      n607 = Round To Nearest(number=w1502) -> (nearest integer value=w1503:dbl)
                      n608 = Divide(x=w1510, y=w1495) -> (x/y=w1506:dbl)
                      n609 = Divide(x=w1505, y=w1495) -> (x/y=w1497:dbl)
                      n610 = Divide(x=w1503, y=w1495) -> (x/y=w1496:dbl)
                      n611 = Bundle(w1506, w1497, w1496) -> (→"I slider 8":cluster{dbl, dbl, dbl})  [unwired: 1 in]
                    }
                    frame 9 {
                      w1515 = 100.0 ("y")
                      n612 = Unbundle By Name(w1514) -> ("Phasor C"=w1527:dbl, "Phasor C"=w1521:dbl, "Phasor C"=w1519:dbl)
                      n613 = Absolute Value(x=w1527) -> (abs(x)=w1528:dbl)
                      n614 = Absolute Value(x=w1521) -> (abs(x)=w1520:dbl)
                      n615 = Absolute Value(x=w1519) -> (abs(x)=w1518:dbl)
                      n616 = Multiply(x=w1528, y=w1515) -> (x*y=w1529:dbl)
                      n617 = Multiply(x=w1520, y=w1515) -> (x*y=w1524:dbl)
                      n618 = Multiply(x=w1518, y=w1515) -> (x*y=w1522:dbl)
                      n619 = Round To Nearest(number=w1529) -> (nearest integer value=w1530:dbl)
                      n620 = Round To Nearest(number=w1524) -> (nearest integer value=w1525:dbl)
                      n621 = Round To Nearest(number=w1522) -> (nearest integer value=w1523:dbl)
                      n622 = Divide(x=w1530, y=w1515) -> (x/y=w1526:dbl)
                      n623 = Divide(x=w1525, y=w1515) -> (x/y=w1517:dbl)
                      n624 = Divide(x=w1523, y=w1515) -> (x/y=w1516:dbl)
                      n625 = Bundle(w1526, w1517, w1516) -> (→"I slider 9":cluster{dbl, dbl, dbl})  [unwired: 1 in]
                    }
                    frame 10 {
                      w1531 = 100.0 ("y")
                      n626 = Unbundle By Name(w1548) -> ("Phasor C"=w1543:dbl, "Phasor C"=w1537:dbl, "Phasor C"=w1535:dbl)
                      n627 = Absolute Value(x=w1543) -> (abs(x)=w1544:dbl)
                      n628 = Absolute Value(x=w1537) -> (abs(x)=w1536:dbl)
                      n629 = Absolute Value(x=w1535) -> (abs(x)=w1534:dbl)
                      n630 = Multiply(x=w1544, y=w1531) -> (x*y=w1545:dbl)
                      n631 = Multiply(x=w1536, y=w1531) -> (x*y=w1540:dbl)
                      n632 = Multiply(x=w1534, y=w1531) -> (x*y=w1538:dbl)
                      n633 = Round To Nearest(number=w1545) -> (nearest integer value=w1546:dbl)
                      n634 = Round To Nearest(number=w1540) -> (nearest integer value=w1541:dbl)
                      n635 = Round To Nearest(number=w1538) -> (nearest integer value=w1539:dbl)
                      n636 = Divide(x=w1546, y=w1531) -> (x/y=w1542:dbl)
                      n637 = Divide(x=w1541, y=w1531) -> (x/y=w1533:dbl)
                      n638 = Divide(x=w1539, y=w1531) -> (x/y=w1532:dbl)
                      n639 = Bundle(w1542, w1533, w1532) -> (→"I slider 10":cluster{dbl, dbl, dbl})  [unwired: 1 in]
                    }
                    frame 11 {
                      w1551 = 100.0 ("y")
                      n640 = Unbundle By Name(w1550) -> ("Phasor C"=w1563:dbl, "Phasor C"=w1557:dbl, "Phasor C"=w1555:dbl)
                      n641 = Absolute Value(x=w1563) -> (abs(x)=w1564:dbl)
                      n642 = Absolute Value(x=w1557) -> (abs(x)=w1556:dbl)
                      n643 = Absolute Value(x=w1555) -> (abs(x)=w1554:dbl)
                      n644 = Multiply(x=w1564, y=w1551) -> (x*y=w1565:dbl)
                      n645 = Multiply(x=w1556, y=w1551) -> (x*y=w1560:dbl)
                      n646 = Multiply(x=w1554, y=w1551) -> (x*y=w1558:dbl)
                      n647 = Round To Nearest(number=w1565) -> (nearest integer value=w1566:dbl)
                      n648 = Round To Nearest(number=w1560) -> (nearest integer value=w1561:dbl)
                      n649 = Round To Nearest(number=w1558) -> (nearest integer value=w1559:dbl)
                      n650 = Divide(x=w1566, y=w1551) -> (x/y=w1562:dbl)
                      n651 = Divide(x=w1561, y=w1551) -> (x/y=w1553:dbl)
                      n652 = Divide(x=w1559, y=w1551) -> (x/y=w1552:dbl)
                      n653 = Bundle(w1562, w1553, w1552) -> (→"I slider 11":cluster{dbl, dbl, dbl})  [unwired: 1 in]
                    }
                    frame 12 {
                      w1569 = 100.0 ("y")
                      n654 = Unbundle By Name(w1568) -> ("Phasor C"=w1581:dbl, "Phasor C"=w1575:dbl, "Phasor C"=w1573:dbl)
                      n655 = Absolute Value(x=w1581) -> (abs(x)=w1582:dbl)
                      n656 = Absolute Value(x=w1575) -> (abs(x)=w1574:dbl)
                      n657 = Absolute Value(x=w1573) -> (abs(x)=w1572:dbl)
                      n658 = Multiply(x=w1582, y=w1569) -> (x*y=w1583:dbl)
                      n659 = Multiply(x=w1574, y=w1569) -> (x*y=w1578:dbl)
                      n660 = Multiply(x=w1572, y=w1569) -> (x*y=w1576:dbl)
                      n661 = Round To Nearest(number=w1583) -> (nearest integer value=w1584:dbl)
                      n662 = Round To Nearest(number=w1578) -> (nearest integer value=w1579:dbl)
                      n663 = Round To Nearest(number=w1576) -> (nearest integer value=w1577:dbl)
                      n664 = Divide(x=w1584, y=w1569) -> (x/y=w1580:dbl)
                      n665 = Divide(x=w1579, y=w1569) -> (x/y=w1571:dbl)
                      n666 = Divide(x=w1577, y=w1569) -> (x/y=w1570:dbl)
                      n667 = Bundle(w1580, w1571, w1570) -> (→"I slider 12":cluster{dbl, dbl, dbl})  [unwired: 1 in]
                    }
                    frame 13 {
                      w1587 = 100.0 ("y")
                      n668 = Unbundle By Name(w1586) -> ("Phasor C"=w1599:dbl, "Phasor C"=w1593:dbl, "Phasor C"=w1591:dbl)
                      n669 = Absolute Value(x=w1599) -> (abs(x)=w1600:dbl)
                      n670 = Absolute Value(x=w1593) -> (abs(x)=w1592:dbl)
                      n671 = Absolute Value(x=w1591) -> (abs(x)=w1590:dbl)
                      n672 = Multiply(x=w1600, y=w1587) -> (x*y=w1601:dbl)
                      n673 = Multiply(x=w1592, y=w1587) -> (x*y=w1596:dbl)
                      n674 = Multiply(x=w1590, y=w1587) -> (x*y=w1594:dbl)
                      n675 = Round To Nearest(number=w1601) -> (nearest integer value=w1602:dbl)
                      n676 = Round To Nearest(number=w1596) -> (nearest integer value=w1597:dbl)
                      n677 = Round To Nearest(number=w1594) -> (nearest integer value=w1595:dbl)
                      n678 = Divide(x=w1602, y=w1587) -> (x/y=w1598:dbl)
                      n679 = Divide(x=w1597, y=w1587) -> (x/y=w1589:dbl)
                      n680 = Divide(x=w1595, y=w1587) -> (x/y=w1588:dbl)
                      n681 = Bundle(w1598, w1589, w1588) -> (→"I slider 13":cluster{dbl, dbl, dbl})  [unwired: 1 in]
                    }
                    frame 14 {
                      w1605 = 100.0 ("y")
                      n682 = Unbundle By Name(w1604) -> ("Phasor C"=w1617:dbl, "Phasor C"=w1611:dbl, "Phasor C"=w1609:dbl)
                      n683 = Absolute Value(x=w1617) -> (abs(x)=w1618:dbl)
                      n684 = Absolute Value(x=w1611) -> (abs(x)=w1610:dbl)
                      n685 = Absolute Value(x=w1609) -> (abs(x)=w1608:dbl)
                      n686 = Multiply(x=w1618, y=w1605) -> (x*y=w1619:dbl)
                      n687 = Multiply(x=w1610, y=w1605) -> (x*y=w1614:dbl)
                      n688 = Multiply(x=w1608, y=w1605) -> (x*y=w1612:dbl)
                      n689 = Round To Nearest(number=w1619) -> (nearest integer value=w1620:dbl)
                      n690 = Round To Nearest(number=w1614) -> (nearest integer value=w1615:dbl)
                      n691 = Round To Nearest(number=w1612) -> (nearest integer value=w1613:dbl)
                      n692 = Divide(x=w1620, y=w1605) -> (x/y=w1616:dbl)
                      n693 = Divide(x=w1615, y=w1605) -> (x/y=w1607:dbl)
                      n694 = Divide(x=w1613, y=w1605) -> (x/y=w1606:dbl)
                      n695 = Bundle(w1616, w1607, w1606) -> (→"I slider 14":cluster{dbl, dbl, dbl})  [unwired: 1 in]
                    }
                    frame 15 {
                      w1623 = 100.0 ("y")
                      n696 = Unbundle By Name(w1622) -> ("Phasor C"=w1635:dbl, "Phasor C"=w1629:dbl, "Phasor C"=w1627:dbl)
                      n697 = Absolute Value(x=w1635) -> (abs(x)=w1636:dbl)
                      n698 = Absolute Value(x=w1629) -> (abs(x)=w1628:dbl)
                      n699 = Absolute Value(x=w1627) -> (abs(x)=w1626:dbl)
                      n700 = Multiply(x=w1636, y=w1623) -> (x*y=w1637:dbl)
                      n701 = Multiply(x=w1628, y=w1623) -> (x*y=w1632:dbl)
                      n702 = Multiply(x=w1626, y=w1623) -> (x*y=w1630:dbl)
                      n703 = Round To Nearest(number=w1637) -> (nearest integer value=w1638:dbl)
                      n704 = Round To Nearest(number=w1632) -> (nearest integer value=w1633:dbl)
                      n705 = Round To Nearest(number=w1630) -> (nearest integer value=w1631:dbl)
                      n706 = Divide(x=w1638, y=w1623) -> (x/y=w1634:dbl)
                      n707 = Divide(x=w1633, y=w1623) -> (x/y=w1625:dbl)
                      n708 = Divide(x=w1631, y=w1623) -> (x/y=w1624:dbl)
                      n709 = Bundle(w1634, w1625, w1624) -> (→"I slider 15":cluster{dbl, dbl, dbl})  [unwired: 1 in]
                    }
                    frame 16 {
                      w1641 = 100.0 ("y")
                      n710 = Unbundle By Name(w1640) -> ("Phasor C"=w1653:dbl, "Phasor C"=w1647:dbl, "Phasor C"=w1645:dbl)
                      n711 = Absolute Value(x=w1653) -> (abs(x)=w1654:dbl)
                      n712 = Absolute Value(x=w1647) -> (abs(x)=w1646:dbl)
                      n713 = Absolute Value(x=w1645) -> (abs(x)=w1644:dbl)
                      n714 = Multiply(x=w1654, y=w1641) -> (x*y=w1655:dbl)
                      n715 = Multiply(x=w1646, y=w1641) -> (x*y=w1650:dbl)
                      n716 = Multiply(x=w1644, y=w1641) -> (x*y=w1648:dbl)
                      n717 = Round To Nearest(number=w1655) -> (nearest integer value=w1656:dbl)
                      n718 = Round To Nearest(number=w1650) -> (nearest integer value=w1651:dbl)
                      n719 = Round To Nearest(number=w1648) -> (nearest integer value=w1649:dbl)
                      n720 = Divide(x=w1656, y=w1641) -> (x/y=w1652:dbl)
                      n721 = Divide(x=w1651, y=w1641) -> (x/y=w1643:dbl)
                      n722 = Divide(x=w1649, y=w1641) -> (x/y=w1642:dbl)
                      n723 = Bundle(w1652, w1643, w1642) -> (→"I slider 16":cluster{dbl, dbl, dbl})  [unwired: 1 in]
                    }
                    frame 17 {
                      w1657 = 100.0 ("y")
                      n724 = Unbundle By Name(w1659) -> ("Phasor C"=w1660:dbl)
                      n725 = Absolute Value(x=w1660) -> (abs(x)=w1661:dbl)
                      n726 = Multiply(x=w1661, y=w1657) -> (x*y=w1662:dbl)
                      n727 = Round To Nearest(number=w1662) -> (nearest integer value=w1663:dbl)
                      n728 = Divide(x=w1663, y=w1657) -> (x/y=→"I slider 17":dbl)
                    }
                    frame 18 {
                      w1664 = 100.0 ("y")
                      n729 = Unbundle By Name(w1666) -> ("Phasor C"=w1667:dbl)
                      n730 = Absolute Value(x=w1667) -> (abs(x)=w1668:dbl)
                      n731 = Multiply(x=w1668, y=w1664) -> (x*y=w1669:dbl)
                      n732 = Round To Nearest(number=w1669) -> (nearest integer value=w1670:dbl)
                      n733 = Divide(x=w1670, y=w1664) -> (x/y=→"I slider 18":dbl)
                    }
                    frame 19 {
                      w1671 = 100.0 ("y")
                      n734 = Unbundle By Name(w1673) -> ("Phasor C"=w1674:dbl)
                      n735 = Absolute Value(x=w1674) -> (abs(x)=w1675:dbl)
                      n736 = Multiply(x=w1675, y=w1671) -> (x*y=w1676:dbl)
                      n737 = Round To Nearest(number=w1676) -> (nearest integer value=w1677:dbl)
                      n738 = Divide(x=w1677, y=w1671) -> (x/y=→"I slider 19":dbl)
                    }
                    frame 20 {
                      w1678 = 100.0 ("y")
                      n739 = Unbundle By Name(w1680) -> ("Phasor C"=w1681:dbl)
                      n740 = Absolute Value(x=w1681) -> (abs(x)=w1682:dbl)
                      n741 = Multiply(x=w1682, y=w1678) -> (x*y=w1683:dbl)
                      n742 = Round To Nearest(number=w1683) -> (nearest integer value=w1684:dbl)
                      n743 = Divide(x=w1684, y=w1678) -> (x/y=→"I slider 20":dbl)
                    }
                    frame 21, Default {
                    }
                  }
                }
              }
            }
            n744 = for {
              tunnel: w703 -> [w714] mode=indexing
              i -> [w713]
              n745 = Unbundle By Name(w714) -> ("Vbus"=w712:cdb[], "Vband"=w709:T4)
              n746 = call "Plot Nodal Voltage.vi"("Range"=w709, "Voltage"=w712) -> ("Vp"=w710:dbl, "Vm"=w711:T9)
              n747 = case shown="True" TRUE {
                tunnel: w711 -> [_ w717]
                tunnel: w713 -> [_ w716]
                tunnel: w710 -> [_ w715]
                frame False {
                }
                frame True {
                  n748 = case shown="18" w716 {
                    tunnel: w717 -> [w725 w733 w741 w749 w757 _ w765 w773 w781 w789 w797 w815 w823 w831 w839 w847 w855 w863 w870 w877 w884 w891 w898 w905 w912 w919 _]
                    tunnel: w715 -> [_ _ _ _ _ _ _ _ _ _ _ _ _ _ _ _ _ _ _ _ _ _ _ _ _ _ _]
                    frame 0 {
                      n749 = Unbundle By Name(w725) -> ("Phasor C"=w724:dbl, "Phasor C"=w719:dbl, "Phasor C"=w718:dbl)
                      n750 = Absolute Value(x=w724) -> (abs(x)=w722:dbl)
                      n751 = Absolute Value(x=w719) -> (abs(x)=w721:dbl)
                      n752 = Absolute Value(x=w718) -> (abs(x)=w720:dbl)
                      n753 = Bundle(w722, w721, w720) -> (→"V slider 0":cluster{dbl, dbl, dbl})  [unwired: 1 in]
                    }
                    frame 1 {
                      n754 = Unbundle By Name(w733) -> ("Phasor C"=w732:dbl, "Phasor C"=w727:dbl, "Phasor C"=w726:dbl)
                      n755 = Absolute Value(x=w732) -> (abs(x)=w730:dbl)
                      n756 = Absolute Value(x=w727) -> (abs(x)=w729:dbl)
                      n757 = Absolute Value(x=w726) -> (abs(x)=w728:dbl)
                      n758 = Bundle(w730, w729, w728) -> (→"V slider 1":cluster{dbl, dbl, dbl})  [unwired: 1 in]
                    }
                    frame 2 {
                      n759 = Unbundle By Name(w741) -> ("Phasor C"=w740:dbl, "Phasor C"=w735:dbl, "Phasor C"=w734:dbl)
                      n760 = Absolute Value(x=w740) -> (abs(x)=w738:dbl)
                      n761 = Absolute Value(x=w735) -> (abs(x)=w737:dbl)
                      n762 = Absolute Value(x=w734) -> (abs(x)=w736:dbl)
                      n763 = Bundle(w738, w737, w736) -> (→"V slider 2":cluster{dbl, dbl, dbl})  [unwired: 1 in]
                    }
                    frame 3 {
                      n764 = Unbundle By Name(w749) -> ("Phasor C"=w748:dbl, "Phasor C"=w743:dbl, "Phasor C"=w742:dbl)
                      n765 = Absolute Value(x=w748) -> (abs(x)=w746:dbl)
                      n766 = Absolute Value(x=w743) -> (abs(x)=w745:dbl)
                      n767 = Absolute Value(x=w742) -> (abs(x)=w744:dbl)
                      n768 = Bundle(w746, w745, w744) -> (→"V slider 3":cluster{dbl, dbl, dbl})  [unwired: 1 in]
                    }
                    frame 4 {
                      n769 = Unbundle By Name(w757) -> ("Phasor C"=w756:dbl, "Phasor C"=w751:dbl, "Phasor C"=w750:dbl)
                      n770 = Absolute Value(x=w756) -> (abs(x)=w754:dbl)
                      n771 = Absolute Value(x=w751) -> (abs(x)=w753:dbl)
                      n772 = Absolute Value(x=w750) -> (abs(x)=w752:dbl)
                      n773 = Bundle(w754, w753, w752) -> (→"V slider 4":cluster{dbl, dbl, dbl})  [unwired: 1 in]
                    }
                    frame 5 {
                    }
                    frame 6 {
                      n774 = Unbundle By Name(w765) -> ("Phasor C"=w764:dbl, "Phasor C"=w759:dbl, "Phasor C"=w758:dbl)
                      n775 = Absolute Value(x=w764) -> (abs(x)=w762:dbl)
                      n776 = Absolute Value(x=w759) -> (abs(x)=w761:dbl)
                      n777 = Absolute Value(x=w758) -> (abs(x)=w760:dbl)
                      n778 = Bundle(w762, w761, w760) -> (→"V slider 6":cluster{dbl, dbl, dbl})  [unwired: 1 in]
                    }
                    frame 7 {
                      n779 = Unbundle By Name(w773) -> ("Phasor C"=w772:dbl, "Phasor C"=w767:dbl, "Phasor C"=w766:dbl)
                      n780 = Absolute Value(x=w772) -> (abs(x)=w770:dbl)
                      n781 = Absolute Value(x=w767) -> (abs(x)=w769:dbl)
                      n782 = Absolute Value(x=w766) -> (abs(x)=w768:dbl)
                      n783 = Bundle(w770, w769, w768) -> (→"V slider 7":cluster{dbl, dbl, dbl})  [unwired: 1 in]
                    }
                    frame 8 {
                      n784 = Unbundle By Name(w781) -> ("Phasor C"=w780:dbl, "Phasor C"=w775:dbl, "Phasor C"=w774:dbl)
                      n785 = Absolute Value(x=w780) -> (abs(x)=w778:dbl)
                      n786 = Absolute Value(x=w775) -> (abs(x)=w777:dbl)
                      n787 = Absolute Value(x=w774) -> (abs(x)=w776:dbl)
                      n788 = Bundle(w778, w777, w776) -> (→"V slider 8":cluster{dbl, dbl, dbl})  [unwired: 1 in]
                    }
                    frame 9 {
                      n789 = Unbundle By Name(w789) -> ("Phasor C"=w788:dbl, "Phasor C"=w783:dbl, "Phasor C"=w782:dbl)
                      n790 = Absolute Value(x=w788) -> (abs(x)=w786:dbl)
                      n791 = Absolute Value(x=w783) -> (abs(x)=w785:dbl)
                      n792 = Absolute Value(x=w782) -> (abs(x)=w784:dbl)
                      n793 = Bundle(w786, w785, w784) -> (→"V slider 9":cluster{dbl, dbl, dbl})  [unwired: 1 in]
                    }
                    frame 10 {
                      n794 = Unbundle By Name(w797) -> ("Phasor C"=w796:dbl, "Phasor C"=w791:dbl, "Phasor C"=w790:dbl)
                      n795 = Absolute Value(x=w796) -> (abs(x)=w794:dbl)
                      n796 = Absolute Value(x=w791) -> (abs(x)=w793:dbl)
                      n797 = Absolute Value(x=w790) -> (abs(x)=w792:dbl)
                      n798 = Bundle(w794, w793, w792) -> (→"V slider 10":cluster{dbl, dbl, dbl})  [unwired: 1 in]
                    }
                    frame 11 {
                      w798 = 10.0 ("y")
                      n799 = Unbundle By Name(w815) -> ("Phasor C"=w814:dbl, "Phasor C"=w812:dbl, "Phasor C"=w811:dbl)
                      n800 = Absolute Value(x=w814) -> (abs(x)=w810:dbl)
                      n801 = Absolute Value(x=w812) -> (abs(x)=w802:dbl)
                      n802 = Absolute Value(x=w811) -> (abs(x)=w801:dbl)
                      n803 = Multiply(x=w810, y=w798) -> (x*y=w809:dbl)
                      n804 = Multiply(x=w802, y=w798) -> (x*y=w806:dbl)
                      n805 = Multiply(x=w801, y=w798) -> (x*y=w804:dbl)
                      n806 = Round To Nearest(number=w809) -> (nearest integer value=w808:dbl)
                      n807 = Round To Nearest(number=w806) -> (nearest integer value=w805:dbl)
                      n808 = Round To Nearest(number=w804) -> (nearest integer value=w803:dbl)
                      n809 = Divide(x=w808, y=w798) -> (x/y=w807:dbl)
                      n810 = Divide(x=w805, y=w798) -> (x/y=w800:dbl)
                      n811 = Divide(x=w803, y=w798) -> (x/y=w799:dbl)
                      n812 = Bundle(w807, w800, w799) -> (→"V slider 11":cluster{dbl, dbl, dbl})  [unwired: 1 in]
                    }
                    frame 12 {
                      n813 = Unbundle By Name(w823) -> ("Phasor C"=w822:dbl, "Phasor C"=w817:dbl, "Phasor C"=w816:dbl)
                      n814 = Absolute Value(x=w822) -> (abs(x)=w820:dbl)
                      n815 = Absolute Value(x=w817) -> (abs(x)=w819:dbl)
                      n816 = Absolute Value(x=w816) -> (abs(x)=w818:dbl)
                      n817 = Bundle(w820, w819, w818) -> (→"V slider 12":cluster{dbl, dbl, dbl})  [unwired: 1 in]
                    }
                    frame 13 {
                      n818 = Unbundle By Name(w831) -> ("Phasor C"=w830:dbl, "Phasor C"=w825:dbl, "Phasor C"=w824:dbl)
                      n819 = Absolute Value(x=w830) -> (abs(x)=w828:dbl)
                      n820 = Absolute Value(x=w825) -> (abs(x)=w827:dbl)
                      n821 = Absolute Value(x=w824) -> (abs(x)=w826:dbl)
                      n822 = Bundle(w828, w827, w826) -> (→"V slider 13":cluster{dbl, dbl, dbl})  [unwired: 1 in]
                    }
                    frame 14 {
                      n823 = Unbundle By Name(w839) -> ("Phasor C"=w838:dbl, "Phasor C"=w833:dbl, "Phasor C"=w832:dbl)
                      n824 = Absolute Value(x=w838) -> (abs(x)=w836:dbl)
                      n825 = Absolute Value(x=w833) -> (abs(x)=w835:dbl)
                      n826 = Absolute Value(x=w832) -> (abs(x)=w834:dbl)
                      n827 = Bundle(w836, w835, w834) -> (→"V slider 14":cluster{dbl, dbl, dbl})  [unwired: 1 in]
                    }
                    frame 15 {
                      n828 = Unbundle By Name(w847) -> ("Phasor C"=w846:dbl, "Phasor C"=w841:dbl, "Phasor C"=w840:dbl)
                      n829 = Absolute Value(x=w846) -> (abs(x)=w844:dbl)
                      n830 = Absolute Value(x=w841) -> (abs(x)=w843:dbl)
                      n831 = Absolute Value(x=w840) -> (abs(x)=w842:dbl)
                      n832 = Bundle(w844, w843, w842) -> (→"V slider 15":cluster{dbl, dbl, dbl})  [unwired: 1 in]
                    }
                    frame 16 {
                      n833 = Unbundle By Name(w855) -> ("Phasor C"=w854:dbl, "Phasor C"=w849:dbl, "Phasor C"=w848:dbl)
                      n834 = Absolute Value(x=w854) -> (abs(x)=w852:dbl)
                      n835 = Absolute Value(x=w849) -> (abs(x)=w851:dbl)
                      n836 = Absolute Value(x=w848) -> (abs(x)=w850:dbl)
                      n837 = Bundle(w852, w851, w850) -> (→"V slider 16":cluster{dbl, dbl, dbl})  [unwired: 1 in]
                    }
                    frame 17 {
                      n838 = Unbundle By Name(w863) -> ("Phasor C"=w862:dbl, "Phasor C"=w857:dbl, "Phasor C"=w856:dbl)
                      n839 = Absolute Value(x=w862) -> (abs(x)=w860:dbl)
                      n840 = Absolute Value(x=w857) -> (abs(x)=w859:dbl)
                      n841 = Absolute Value(x=w856) -> (abs(x)=w858:dbl)
                      n842 = Bundle(w860, w859, w858) -> (→"V slider 17":cluster{dbl, dbl, dbl})  [unwired: 1 in]
                    }
                    frame 18 {
                      w866 = 10.0 ("y")
                      n843 = Unbundle By Name(w870) -> ("Phasor C"=w869:dbl)
                      n844 = Absolute Value(x=w869) -> (abs(x)=w865:dbl)
                      n845 = Multiply(x=w865, y=w866) -> (x*y=w868:dbl)
                      n846 = Round To Nearest(number=w868) -> (nearest integer value=w867:dbl)
                      n847 = Divide(x=w867, y=w866) -> (x/y=→"V slider 18":dbl)
                    }
                    frame 19 {
                      w873 = 10.0 ("y")
                      n848 = Unbundle By Name(w877) -> ("Phasor C"=w876:dbl)
                      n849 = Absolute Value(x=w876) -> (abs(x)=w872:dbl)
                      n850 = Multiply(x=w872, y=w873) -> (x*y=w875:dbl)
                      n851 = Round To Nearest(number=w875) -> (nearest integer value=w874:dbl)
                      n852 = Divide(x=w874, y=w873) -> (x/y=→"V slider 19":dbl)
                    }
                    frame 20 {
                      w880 = 10.0 ("y")
                      n853 = Unbundle By Name(w884) -> ("Phasor C"=w883:dbl)
                      n854 = Absolute Value(x=w883) -> (abs(x)=w879:dbl)
                      n855 = Multiply(x=w879, y=w880) -> (x*y=w882:dbl)
                      n856 = Round To Nearest(number=w882) -> (nearest integer value=w881:dbl)
                      n857 = Divide(x=w881, y=w880) -> (x/y=→"V slider 20":dbl)
                    }
                    frame 21 {
                      w887 = 10.0 ("y")
                      n858 = Unbundle By Name(w891) -> ("Phasor C"=w890:dbl)
                      n859 = Absolute Value(x=w890) -> (abs(x)=w886:dbl)
                      n860 = Multiply(x=w886, y=w887) -> (x*y=w889:dbl)
                      n861 = Round To Nearest(number=w889) -> (nearest integer value=w888:dbl)
                      n862 = Divide(x=w888, y=w887) -> (x/y=→"V slider 21":dbl)
                    }
                    frame 22 {
                      w894 = 10.0 ("y")
                      n863 = Unbundle By Name(w898) -> ("Phasor C"=w897:dbl)
                      n864 = Absolute Value(x=w897) -> (abs(x)=w893:dbl)
                      n865 = Multiply(x=w893, y=w894) -> (x*y=w896:dbl)
                      n866 = Round To Nearest(number=w896) -> (nearest integer value=w895:dbl)
                      n867 = Divide(x=w895, y=w894) -> (x/y=→"V slider 22":dbl)
                    }
                    frame 23 {
                      w901 = 10.0 ("y")
                      n868 = Unbundle By Name(w905) -> ("Phasor C"=w904:dbl)
                      n869 = Absolute Value(x=w904) -> (abs(x)=w900:dbl)
                      n870 = Multiply(x=w900, y=w901) -> (x*y=w903:dbl)
                      n871 = Round To Nearest(number=w903) -> (nearest integer value=w902:dbl)
                      n872 = Divide(x=w902, y=w901) -> (x/y=→"V slider 23":dbl)
                    }
                    frame 24 {
                      w908 = 10.0 ("y")
                      n873 = Unbundle By Name(w912) -> ("Phasor C"=w911:dbl)
                      n874 = Absolute Value(x=w911) -> (abs(x)=w907:dbl)
                      n875 = Multiply(x=w907, y=w908) -> (x*y=w910:dbl)
                      n876 = Round To Nearest(number=w910) -> (nearest integer value=w909:dbl)
                      n877 = Divide(x=w909, y=w908) -> (x/y=→"V slider 24":dbl)
                    }
                    frame 25 {
                      w915 = 10.0 ("y")
                      n878 = Unbundle By Name(w919) -> ("Phasor C"=w918:dbl)
                      n879 = Absolute Value(x=w918) -> (abs(x)=w914:dbl)
                      n880 = Multiply(x=w914, y=w915) -> (x*y=w917:dbl)
                      n881 = Round To Nearest(number=w917) -> (nearest integer value=w916:dbl)
                      n882 = Divide(x=w916, y=w915) -> (x/y=→"V slider 25":dbl)
                    }
                    frame 26, Default {
                    }
                  }
                }
              }
            }
          }
          frame True {
          }
        }
        n883 = Wait on Notification(notifier=w699, timeout in ms (-1)=w693, error in (no error)=w697) -> (notifier out=w698:refnum<notifier>, notification=w692:bool, error out=w696:errorcluster)  [unwired: 1 in, 1 out]
        n884 = local write "Stop?"(w692) -> ()
        n885 = Wait (ms)(milliseconds to wait=u32 5) -> ()  [unwired: 1 out]
      }
      n886 = UDP Open(8:w670, 11:u16 54321 ("port")) -> (port=w673:refnum<k16>, 0:w671:errorcluster)  [unwired: 3 in, 1 out]
      n887 = while {
        shift-right: [w683] -> w672
        shift-left: w671 -> [w690]
        shift-right: [w687] -> w674
        shift-left: w673 -> [w689]
        stop <- "Stop?" stop-if-true
        # "Receive"
        n888 = UDP Read(connection ID=w689, timeout ms (25000)=-1, 8:w690) -> (data out=w686:string, error out=w684:errorcluster, 3:w687:refnum<k16>)  [unwired: 1 in, 2 out]
        n889 = Unflatten From JSON(JSON string=w686, type and defaults=cluster{"Connected?":bool} {"Connected?"=TRUE}, error in (no error)=w684) -> (value=w681:cluster{"Connected?":bool}, error out=w683:errorcluster)  [unwired: 4 in]
        n890 = Unbundle By Name(w681) -> ("Connected?"=→"Connected?":bool)
      }
      n891 = UDP Close(connection ID=w674, 8:w672) -> (error out=w667:errorcluster)  [unwired: 1 out]
      n892 = Merge Errors(w669, w667) -> (w668:errorcluster)
    }
  }
  "Stop (Out)" <- w9
  "Error (Out)" <- w4
  "SCADA AugState (Out)" <- w2
